vi "MegaAwesome_8_30_12a_JW.vi"() -> ()   [LabVIEW 2011]
uses:
  MegaAwesome_States.ctl
  <vilib>/Utility/file.llb/Read From Spreadsheet File (string).vi
  <vilib>/Utility/file.llb/Write To Spreadsheet File (string).vi
panel:
  in  "Slider Min":dbl=5.0
  in  "Slider Max":dbl=5.0
  out "Opj X Axis":string
  out "X Axis Display Type":string
  in  "Index-Sat":dbl=5.0
  in  "Index-Lin":dbl=5.0
  in  "IndexLog-Lin":dbl=5.0
  in  "IndexLog-Sat":dbl=5.0 caption="Num Pts"
  out "Lin Id-Log Used":dbl[](array[numeric])
  out "Lin-Vg Array-Log Used":dbl[](array[numeric])
  out "Total Width":dbl
  in  "New: Comments":string
  out "Save Array":string[][](array[string])
  out "Folder Index":i32 caption="Length"
  out "Sat Id-Used":dbl[](array[numeric])
  out "Sat Vg Array-Used":dbl[](array[numeric])
  out "Vg Array-Log-Used":dbl[](array[numeric])
  out "Sat Id-Log-Used":dbl[](array[numeric])
  out "Lin Id-Used":dbl[](array[numeric])
  out "Lin-Vg Array-Used":dbl[](array[numeric])
  out "Lin Vd":dbl
  out "Recorded Prop":T1
  out "Current State":T2
  in  "Main Tab Control":T3(tab)
  in  "Image Folder":path
  out "Image File":path=path "D:/UserData/Desktop/Jeremy/WFU/Research/Programs/VI mods/Image Not Found.png"
  in  "Transfer File":path
  out "Transfer Folder":path
  out "Fabrication Prop":T4
  in  "Transfer Plots":T5(tab)=enum."Saturation"
  in  "Lin-Trans Slider":dbl(slide) step=1.0 scale=-40.0..40.0 scale format="%#_1p"
  out "Sqrt-Lin":cluster{dbl[], dbl[]}[](graph)
  in  "Sat-Trans Slider":dbl(slide) step=1.0 scale=-40.0..40.0 scale format="%#_1p"
  out "Sqrt-Sat":cluster{dbl[], dbl[]}[](graph)
  out "Raw- Lin":cluster{dbl[], dbl[]}[](graph)
  out "Raw- Sat":cluster{dbl[], dbl[]}[](graph)
  in  "Log Plots":enum32{"Linear", "Saturation", "Transport"}(tab)=enum."Saturation"
  in  "Lin-Log Slider":dbl(slide) step=1.0 scale=-40.0..40.0 scale format="%#_1p"
  out "Log-Lin":cluster{dbl[], dbl[]}[](graph)
  in  "Sat-Log Slider":dbl(slide) step=1.0 scale=-40.0..40.0 scale format="%#_1p"
  out "Sat-Log":cluster{dbl[], dbl[]}[](graph)
  out "Transport":cluster{dbl[], dbl[]}[](graph)
  in  "Manual Controls":T6
  in  "File Controls":T7
  out "Date Recorded":string="Date Recorded" caption="Measured"
  out "Data Name:":string
  out "Image Name":string
  out "Index":string
  out "Date Created":string caption="Fabricated"
  in  "Comments:":string
  out "Rec: Length":dbl caption="Length" format="%#_3g"
  out "Rec: Width":dbl caption="Width" format="%#_4g"
  out "Rec: Dielectric (d)":dbl caption="Dielectric (d)" format="%#_3g"
  in  "New: Dielectric":dbl
  in  "New: Length":dbl
  in  "New: Width":dbl
  out "Rec: Temp":dbl caption="Sample Temp" format="%.1f"
  in  "New: Temp":dbl format="%.1f"
  out "Image Out":T8(plugin-control)
  in  "Num Pts":dbl=5.0
  in  "Num Pts Log":dbl=5.0 caption="Num Pts"
  out "Recorded Values Cluster":T9
  out "Calculated Values Cluster":T9 caption="Recorded Values Cluster"
  out "Re-Calculated Values Cluster":T9 caption="Recorded Values Cluster"
  in  "Independant Variable:":string(combo)="Length (um):"
  out "Image Preview":T8(plugin-control)
  in  "No Image File":path=path "\\\\acad1\\physics/Jurchescu-group/JW-PD/Mega Awesome/Image Not Found.png"
  in  "Room Temp":dbl=294.0
  in  "Origin Project File":path=path "\\\\acad1\\physics/Jurchescu-group/JW-PD/Group Library/Origin Project Files/DeviceData_8_10_12a_JW.opj"
  in  "Transport Style Controls":T10={"Transport Line Size"=1, "Transport Line Color"=16772608} {"Transport Line Size" items=["Extra Small", "Small", "Medium", "Large", "Extra Large"]}
  # "Image Location"
  # "Recorded"
  # "Calculated"
  # "Re-Calculated"
  # "Manual"
  # "Used points display at y=0\nValues are wrong w/ slider"
  # "Slider\nDoesn't\nWork"
  # "Slider\nDoesn't\nWork"
  # "No new points displayed"
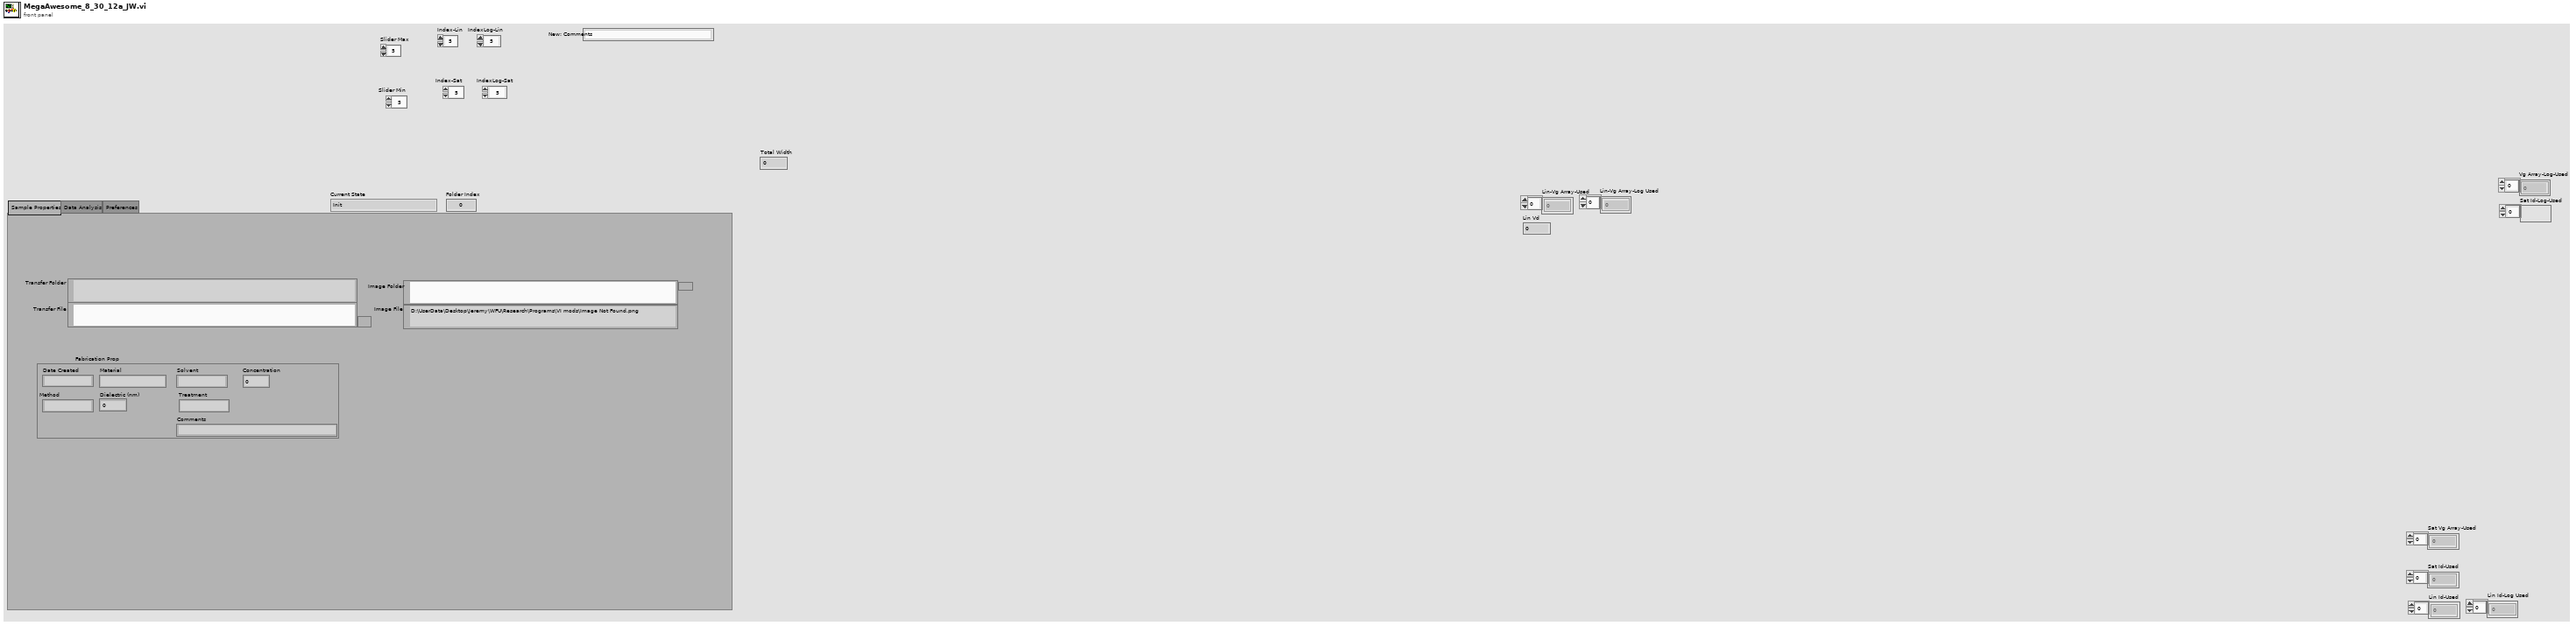
[diagram p1: front panel]
types:
  T1 = cluster{"Date Recorded":string, "Index":string, "Length":dbl, "Width":dbl, "Sample Temp":dbl}
  T2 = typedef "MegaAwesome_States.ctl" = enum16{"Init", "File Missing", "No Event", "Read Data", "Calculated Values", "Re-Calculated Values", "Next File", "Previous File", "Discard File", "Save", "Save Lines", "Export", "Exit"}
  T3 = enum32{"Sample Properties", "Data Analysis", "Preferences"}
  T4 = cluster{"Date Created":string, "Material":string, "Solvent":string, "Concentration":dbl, "Method":string, "Dielectric (nm)":dbl, "Treatment":string, "Comments":string}
  T5 = enum32{"Linear", "Saturation", "Raw-Linear", "Raw-Saturation"}
  T6 = cluster{"Manual-Temp":bool, "Manual-Width":bool, "Manuel-Length":bool, "Manuel-Dielectric":bool, "Manual Comments":bool}
  T7 = cluster{"Previous File":bool, "Discard ":bool, "Save Lines":bool, "Close":bool, "Next File ":bool, "Save":bool, "Save Next":bool, "Export":bool}
  T8 = typedef "IMAQ Image.ctl" = refnum<image>
  T9 = cluster{"Mobility-Sat":dbl, "Moblitity-Lin":dbl, "On/Off":dbl, "Off Current":dbl, "Vt-Sat":dbl, "STS":dbl, "Trap Density-VT":dbl, "Trap Density-STS":dbl}
  T10 = cluster{"Transport Line Size":u16, "Transport Line Color":u32}
  T11 = cluster{"[0]":cluster{dbl[], dbl[]}, "[1]":cluster{dbl[], dbl[]}, "[2]":cluster{dbl[], dbl[]}, "[3]":cluster{dbl[], dbl[]}, "[4]":cluster{dbl[], dbl[]}, "[5]":cluster{dbl[], dbl[]}, "[6]":cluster{dbl[], dbl[]}, "[7]":cluster{dbl[], dbl[]}, "[8]":cluster{dbl[], dbl[]}}
  T12 = cluster{"Sat Vg Used":dbl[], "Sat Sqrt(Id) Used ":dbl[], "Lin Vg Used":dbl[], "Lin Sqrt(Id) Used":dbl[], "Index-Lin":dbl, "Index-Sat":dbl}
  T13 = cluster{"Raw Sat":cluster{dbl[], dbl[]}[], "Sqrt Sat":cluster{dbl[], dbl[]}[], "Log Sat":cluster{dbl[], dbl[]}[], "Raw Lin":cluster{dbl[], dbl[]}[], "Sqrt Lin":cluster{dbl[], dbl[]}[], "Log Lin":cluster{dbl[], dbl[]}[]}
  T14 = cluster{"Mobility-Sat":dbl, "Vt-Sat":dbl, "Mobility-Lin":dbl, "Vt-Lin":dbl, "Off I-Sat":dbl, "On/Off I-Sat":dbl}
  T15 = cluster{"Sat Vg Used":dbl[], "Sat Log(Id) Used":dbl[], "Lin Vg Used":dbl[], "Lin Log(Id) Used":dbl[], "STS Index-Sat":dbl, "STS Index-Lin":dbl}
  T16 = cluster{"Independant  Variable Indicator":string, "Parameter String Indicator":string}
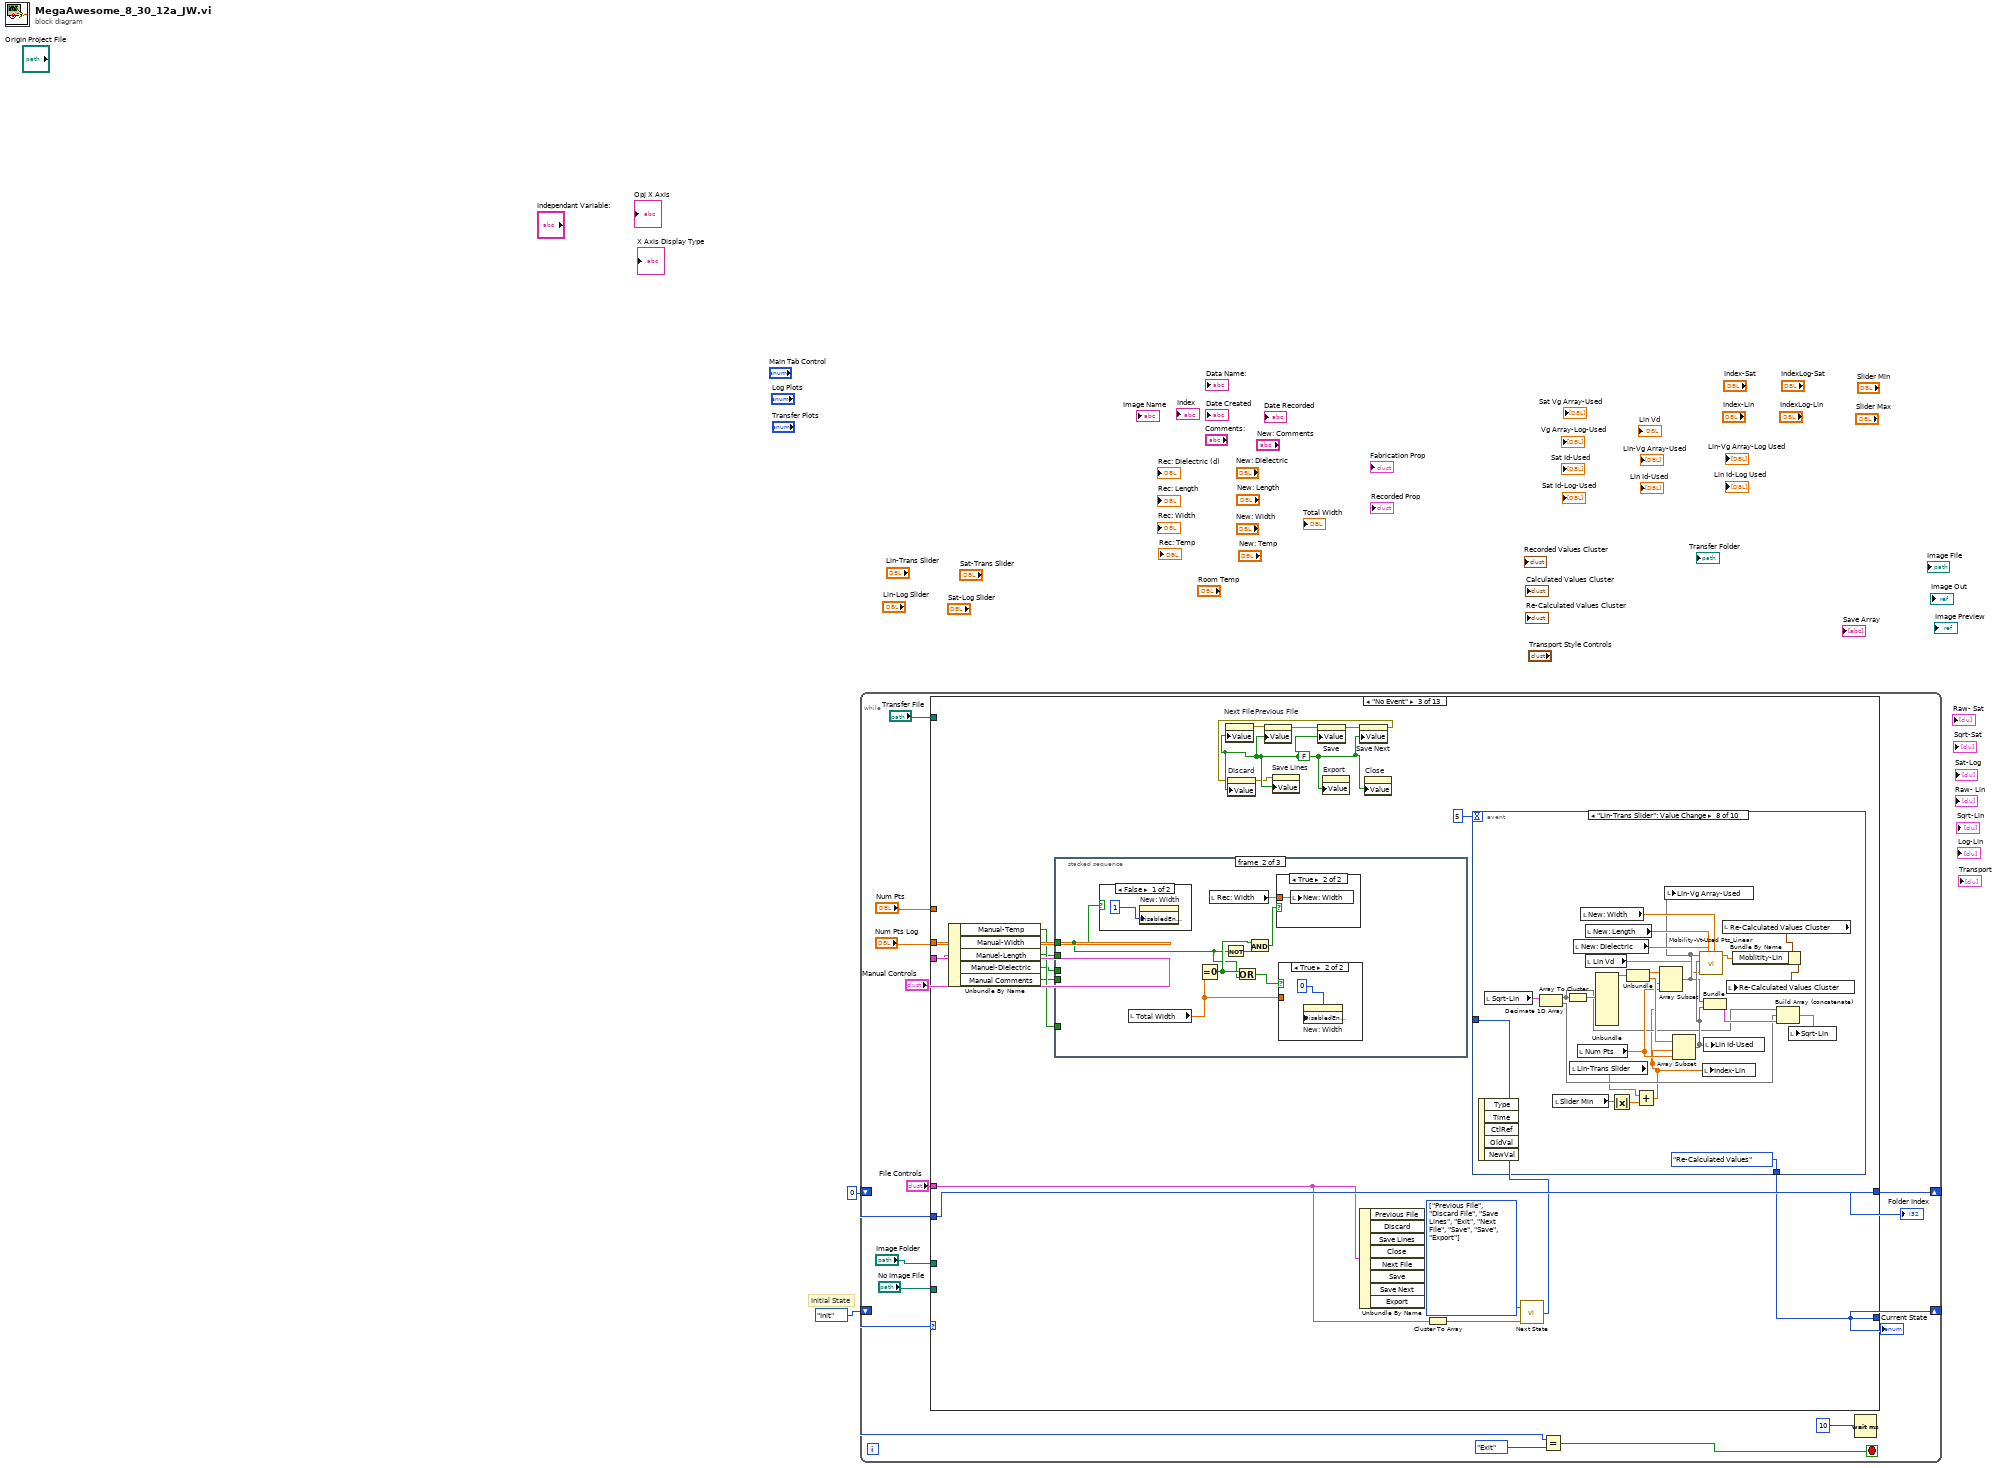
[diagram p0: block diagram]
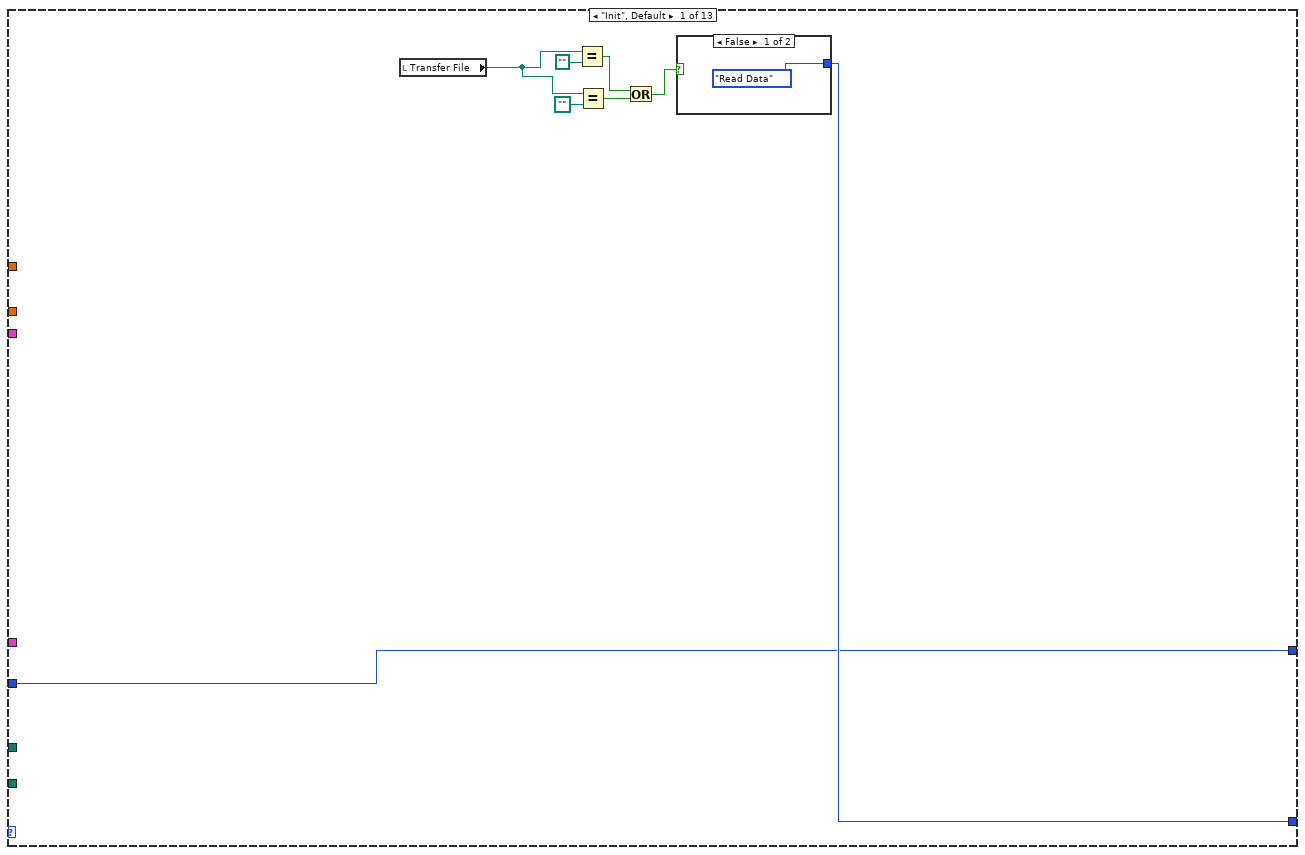
[diagram p2: hidden frame]
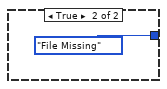
[diagram p3: hidden frame]
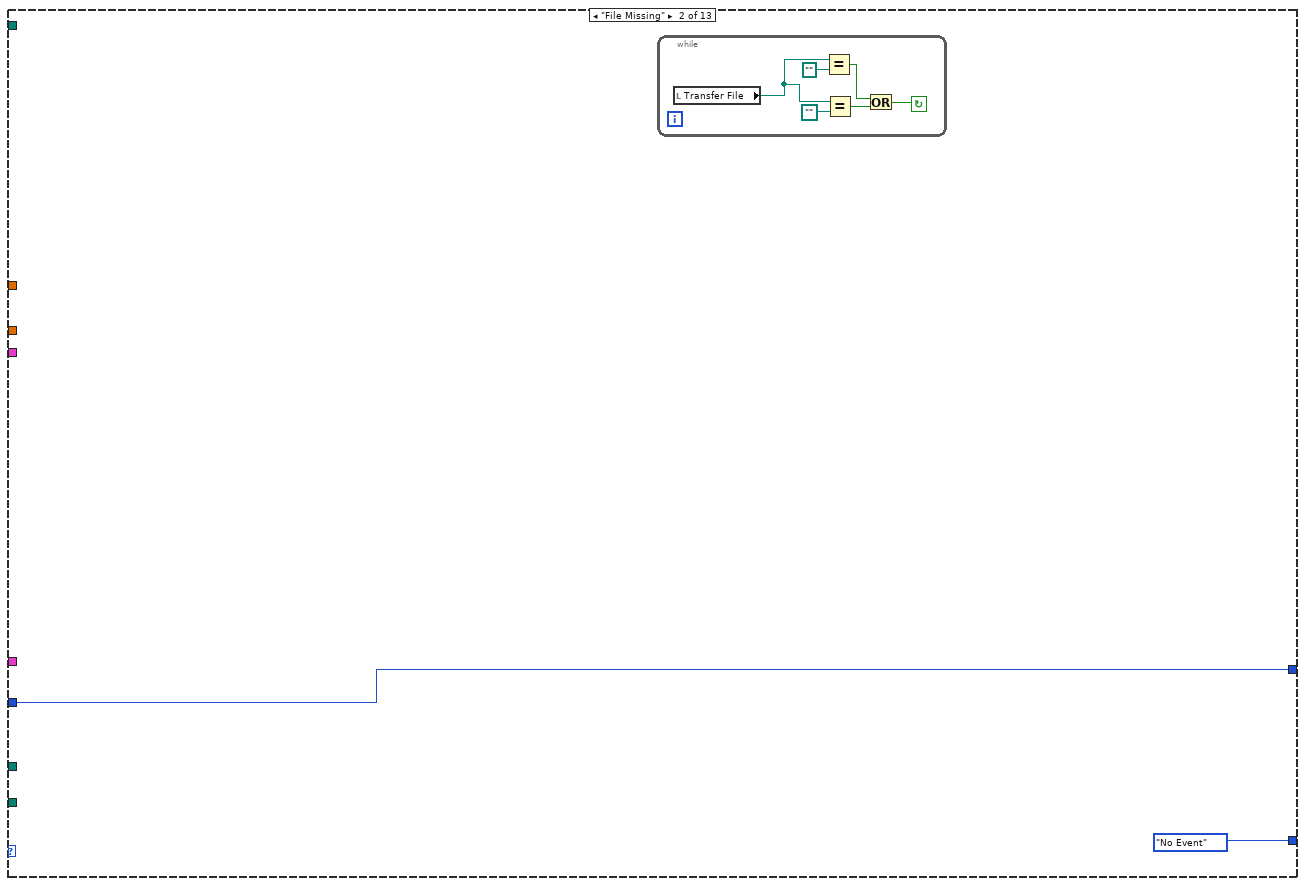
[diagram p4: hidden frame]
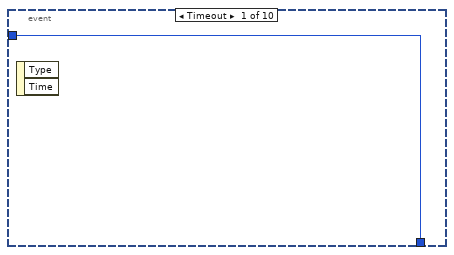
[diagram p5: hidden frame]
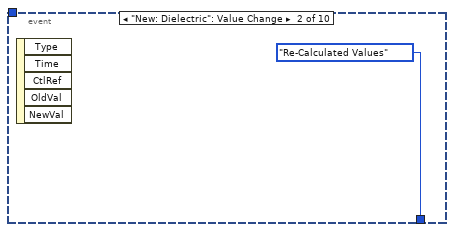
[diagram p6: hidden frame]
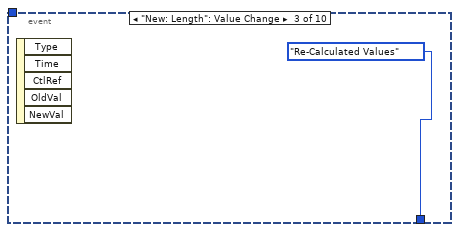
[diagram p7: hidden frame]
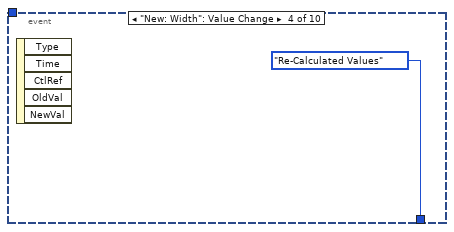
[diagram p8: hidden frame]
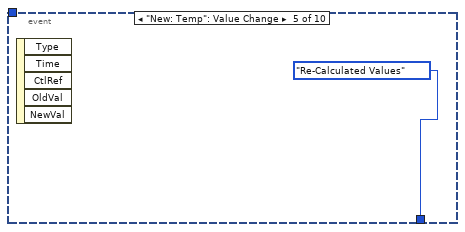
[diagram p9: hidden frame]
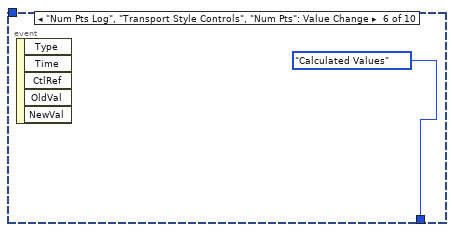
[diagram p10: hidden frame]
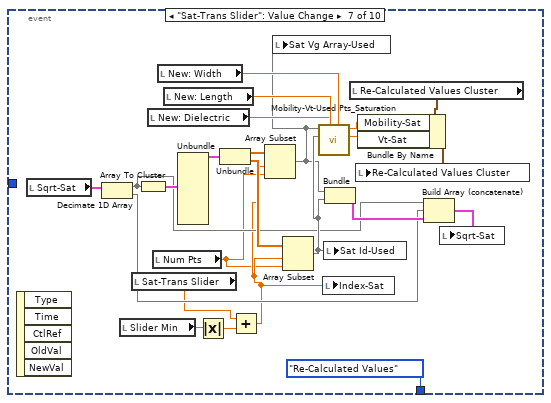
[diagram p11: hidden frame]
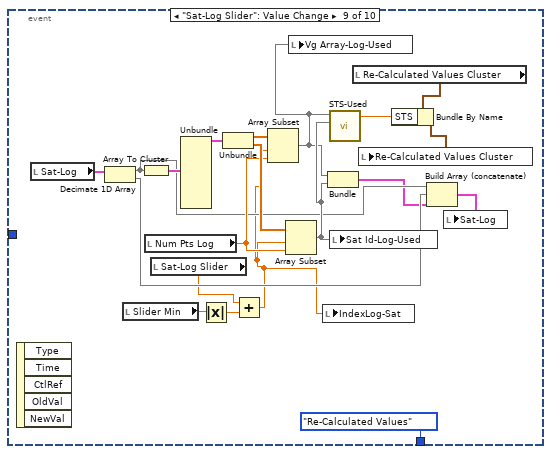
[diagram p12: hidden frame]
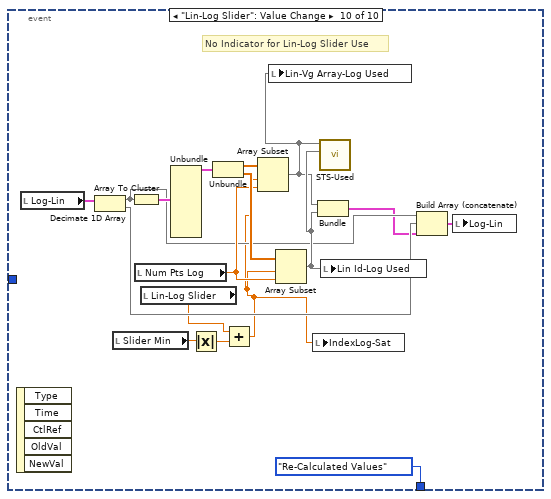
[diagram p13: hidden frame]
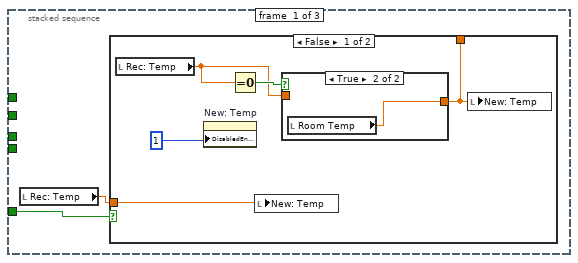
[diagram p14: hidden frame]
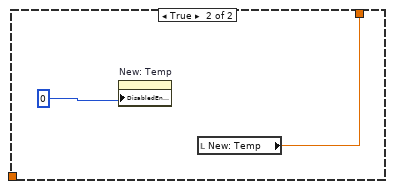
[diagram p16: hidden frame]
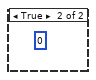
[diagram p17: hidden frame]
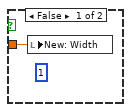
[diagram p19: hidden frame]
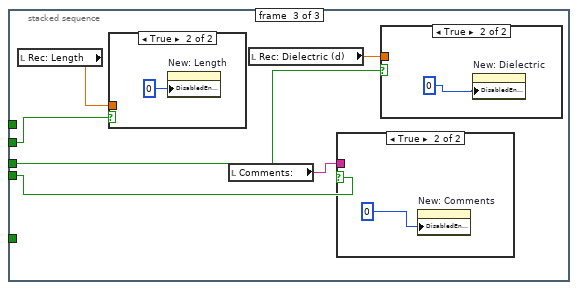
[diagram p20: hidden frame]
diagram:
  # "Initial State"
  n1 = while {
    shift-right: [w13] -> _
    shift-left: MegaAwesome_States."Init" -> [w15]
    shift-right: [w6] -> _
    shift-left: 0 -> [w7]
    stop <- w16 stop-if-true
    n2 = case shown="\"No Event\"" w15 {
      tunnel: [w18 MegaAwesome_States."No Event" w43 MegaAwesome_States."Calculated Values" MegaAwesome_States."Re-Calculated Values" MegaAwesome_States."No Event" MegaAwesome_States."Read Data" MegaAwesome_States."Read Data" MegaAwesome_States."No Event" w341 MegaAwesome_States."No Event" MegaAwesome_States."No Event" MegaAwesome_States."Exit"] -> w13
      tunnel: "Transfer File" -> [_ _ _ w188 w225 _ w310 w322 _ w346 _ _ _]
      tunnel: "Num Pts" -> [_ _ _ _ w249 _ _ _ _ _ _ _ _]
      tunnel: "Num Pts Log" -> [_ _ _ _ w248 _ _ _ _ _ _ _ _]
      tunnel: "Image Folder" -> [_ _ _ _ w245 _ _ _ _ _ _ _ _]
      tunnel: "No Image File" -> [_ _ _ _ w244 _ _ _ _ _ _ _ _]
      tunnel: [w17 w27 w51 w182 w243 w270 w295 w320 w338 w347 w862 w865 w866] -> w6
      tunnel: w7 -> [w17 w27 w51 _ w243 w270 w296 w321 w338 w347 w862 w865 w866]
      tunnel: "Manual Controls" -> [_ _ w45 _ _ _ _ _ _ w345 _ _ _]
      tunnel: "File Controls" -> [_ _ w41 _ _ _ _ _ _ w340 _ _ _]
      frame "Init", Default {
        n3 = local read "Transfer File"() -> (w19:path)
        n4 = Equal?(x=w19, y=path "") -> (x = y?=w22:bool)
        n5 = Equal?(x=w19, y=path "") -> (x = y?=w21:bool)
        n6 = Or(x=w22, y=w21) -> (x .or. y?=w24:bool)
        n7 = case shown="False" w24 {
          tunnel: [MegaAwesome_States."Read Data" MegaAwesome_States."File Missing"] -> w18
          frame False {
          }
          frame True {
          }
        }
      }
      frame "File Missing" {
        n8 = while {
          stop <- w29 continue-if-true
          n9 = local read "Transfer File"() -> (w30:path)
          n10 = Equal?(x=w30, y=path "") -> (x = y?=w32:bool)
          n11 = Equal?(x=w30, y=path "") -> (x = y?=w33:bool)
          n12 = Or(x=w32, y=w33) -> (x .or. y?=w29:bool)
        }
      }
      frame "No Event" {
        w40 = FALSE
        w53 = T2[] [enum."Previous File", enum."Discard File", enum."Save Lines", enum."Exit", enum."Next File", enum."Save", enum."Save", enum."Export"] items=["Init", "File Missing", "No Event", "Read Data", "Calculated Values", "Re-Calculated Values", "Next File", "Previous File", "Discard File", "Save", "Save Lines", "Export", "Exit"]
        n13 = Unbundle By Name(w45) -> ("Manual-Temp"=w50:bool, "Manual-Width"=w49:bool, "Manuel-Length"=w48:bool, "Manuel-Dielectric"=w47:bool, "Manual Comments"=w46:bool)
        n14 = stacked-sequence {
          tunnel: w50 -> [w146 _ _]
          tunnel: w49 -> [_ w156 _]
          tunnel: w48 -> [_ _ w171]
          tunnel: w47 -> [_ _ w168]
          tunnel: w46 -> [_ _ w167]
          frame #0 {
            n15 = local read "Rec: Temp"() -> (w145:dbl)
            n16 = case shown="False" w146 {
              tunnel: w145 -> [w151 _]
              tunnel: [w148 w155] -> _
              frame False {
                n17 = local read "Rec: Temp"() -> (w149:dbl)
                n18 = property on="New: Temp" class="DigNum (strict)"("DisabledEnum"=1) -> ()  [unwired: 2 in, 2 out]
                n19 = Equal To 0?(x=w149) -> (x = 0?=w150:bool)
                n20 = local write "New: Temp"(w151) -> ()
                n21 = case shown="True" w150 {
                  tunnel: [w152 w153] -> w148
                  tunnel: w149 -> [w152 _]
                  frame False {
                  }
                  frame True {
                    n22 = local read "Room Temp"() -> (w153:dbl)
                  }
                }
                n23 = local write "New: Temp"(w148) -> ()
              }
              frame True {
                n24 = property on="New: Temp" class="DigNum (strict)"("DisabledEnum"=0) -> ()  [unwired: 2 in, 2 out]
                n25 = local read "New: Temp"() -> (w155:dbl)
              }
            }
          }
          frame #1 {
            n26 = case shown="False" w156 {
              frame False {
                n27 = property on="New: Width" class="DigNum (strict)"("DisabledEnum"=1) -> ()  [unwired: 2 in, 2 out]
              }
              frame True {
                (unwired) 0
              }
            }
            n28 = local read "Total Width"() -> (w162:dbl)
            n29 = Equal To 0?(x=w162) -> (x = 0?=w159:bool)
            n30 = local read "Rec: Width"() -> (w160:dbl)
            n31 = Not(x=w156) -> (.not. x?=w158:bool)
            n32 = Or(x=w159, y=w156) -> (x .or. y?=w161:bool)
            n33 = And(x=w159, y=w158) -> (x .and. y?=w157:bool)
            n34 = case shown="True" w157 {
              tunnel: w160 -> [_ w164]
              frame False {
              }
              frame True {
                n35 = local write "New: Width"(w164) -> ()
              }
            }
            n36 = case shown="True" w161 {
              tunnel: w162 -> [w165 _]
              frame False {
                (unwired) 1
                n37 = local write "New: Width"(w165) -> ()
              }
              frame True {
                n38 = property on="New: Width" class="DigNum (strict)"("DisabledEnum"=0) -> ()  [unwired: 2 in, 2 out]
              }
            }
          }
          frame #2 {
            n39 = local read "Rec: Length"() -> (w172:dbl)
            n40 = case shown="True" w171 {
              tunnel: w172 -> [w180 _]
              frame False {
                n41 = local write "New: Length"(w180) -> ()
                n42 = property on="New: Length" class="DigNum (strict)"("DisabledEnum"=1) -> ()  [unwired: 2 in, 2 out]
              }
              frame True {
                n43 = property on="New: Length" class="DigNum (strict)"("DisabledEnum"=0) -> ()  [unwired: 2 in, 2 out]
              }
            }
            n44 = local read "Comments:"() -> (w169:string)
            n45 = local read "Rec: Dielectric (d)"() -> (w170:dbl)
            n46 = case shown="True" w167 {
              tunnel: w169 -> [w174 _]
              frame False {
                n47 = local write "New: Comments"(w174) -> ()
                n48 = property on="New: Comments" class="Str"("DisabledEnum"=1) -> ()  [unwired: 2 in, 2 out]
              }
              frame True {
                n49 = property on="New: Comments" class="Str"("DisabledEnum"=0) -> ()  [unwired: 2 in, 2 out]
              }
            }
            n50 = case shown="True" w168 {
              tunnel: w170 -> [w177 _]
              frame False {
                n51 = local write "New: Dielectric"(w177) -> ()
                n52 = property on="New: Dielectric" class="DigNum (strict)"("DisabledEnum"=1) -> ()  [unwired: 2 in, 2 out]
              }
              frame True {
                n53 = property on="New: Dielectric" class="DigNum (strict)"("DisabledEnum"=0) -> ()  [unwired: 2 in, 2 out]
              }
            }
          }
        }
        n54 = property on="Next File" class="Bool (strict)"("Value"=w40) -> (error out=w39:errorcluster)  [unwired: 2 in, 1 out]
        n55 = property on="Previous File" class="Bool (strict)"(error in=w39, "Value"=w40) -> (error out=w38:errorcluster)  [unwired: 1 in, 1 out]
        n56 = property on="Save" class="Bool (strict)"(error in=w38, "Value"=w40) -> (error out=w37:errorcluster)  [unwired: 1 in, 1 out]
        n57 = property on="Export" class="Bool (strict)"("Value"=w40) -> ()  [unwired: 2 in, 2 out]
        n58 = Unbundle By Name(w41) -> ()  [unwired: 8 out]
        n59 = property on="Save Next" class="Bool (strict)"(error in=w37, "Value"=w40) -> (error out=w36:errorcluster)  [unwired: 1 in, 1 out]
        n60 = property on="Discard" class="Bool (strict)"(error in=w36, "Value"=w40) -> (error out=w35:errorcluster)  [unwired: 1 in, 1 out]
        n61 = property on="Save Lines" class="Bool (strict)"(error in=w35, "Value"=w40) -> ()  [unwired: 1 in, 2 out]
        n62 = property on="Close" class="Bool (strict)"("Value"=w40) -> ()  [unwired: 2 in, 2 out]
        n63 = Cluster To Array(cluster=w41) -> (array=w52:bool[])
        n64 = call "Next State.vi"("Buttons []"=w52, "States []"=w53) -> ("Enum"=w44:T2)
        n65 = event shown="[7] \"Lin-Trans Slider\": Value Change" {
          selector: _ -> [_ _ _ _ _ _ _ _ _ _]
          dyn-events: _ -> [_ _ _ _ _ _ _ _ _ _]
          timeout: 5 -> [_ _ _ _ _ _ _ _ _ _]
          tunnel: w44 -> [w54 _ _ _ _ _ _ _ _ _]
          tunnel: [w54 MegaAwesome_States."Re-Calculated Values" MegaAwesome_States."Re-Calculated Values" MegaAwesome_States."Re-Calculated Values" MegaAwesome_States."Re-Calculated Values" MegaAwesome_States."Calculated Values" MegaAwesome_States."Re-Calculated Values" MegaAwesome_States."Re-Calculated Values" MegaAwesome_States."Re-Calculated Values" MegaAwesome_States."Re-Calculated Values"] -> w43
          event Timeout {
            n66 = event-data() -> ()  [unwired: 1 in, 2 out]
          }
          event "New: Dielectric": Value Change {
            n67 = event-data() -> ()  [unwired: 1 in, 5 out]
          }
          event "New: Length": Value Change {
            n68 = event-data() -> ()  [unwired: 1 in, 5 out]
          }
          event "New: Width": Value Change {
            n69 = event-data() -> ()  [unwired: 1 in, 5 out]
          }
          event "New: Temp": Value Change {
            n70 = event-data() -> ()  [unwired: 1 in, 5 out]
          }
          event "Num Pts Log", "Transport Style Controls", "Num Pts": Value Change {
            n71 = event-data() -> ()  [unwired: 1 in, 5 out]
          }
          event "Sat-Trans Slider": Value Change {
            n72 = event-data() -> ()  [unwired: 1 in, 5 out]
            n73 = local read "Sqrt-Sat"() -> (w83:cluster{dbl[], dbl[]}[])
            n74 = Decimate 1D Array(w83) -> (w67:cluster{dbl[], dbl[]}[], w68:cluster{dbl[], dbl[]}[])
            n75 = local read "Slider Min"() -> (w64:dbl)
            n76 = local read "Sat-Trans Slider"() -> (w62:dbl)
            n77 = Array To Cluster(array=w67) -> (cluster=w82:T11)
            n78 = local read "New: Dielectric"() -> (w77:dbl)
            n79 = local read "Num Pts"() -> (w60:dbl)
            n80 = local read "New: Width"() -> (w79:dbl)
            n81 = local read "New: Length"() -> (w78:dbl)
            n82 = Unbundle(w82) -> ("[0]"=w81:cluster{dbl[], dbl[]})  [unwired: 8 out]
            n83 = Absolute Value(x=w64) -> (abs(x)=w63:dbl)
            n84 = Unbundle(w81) -> (w65:dbl[], w80:dbl[])
            n85 = Add(x=w62, y=w63) -> (x+y=w61:dbl)
            n86 = Array Subset(array=w65, index=w61, length=w60) -> (w75:dbl[])
            n87 = local write "Sat Vg Array-Used"(w75) -> ()
            n88 = Array Subset(array=w80, index=w61, length=w60) -> (w76:dbl[])
            n89 = call "Mobility-Vt-Used Pts_Saturation.vi"("Width"=w79, "Length"=w78, "Dielectric (d)"=w77, "Sat Id Used"=w76, "Vg Used"=w75) -> ("Vt"=w71:dbl, "Mobility"=w72:dbl)  [unwired: 4 in, 1 out]
            n90 = local write "Index-Sat"(w61) -> ()
            n91 = local write "Sat Id-Used"(w76) -> ()
            n92 = Bundle(w75, w76) -> (w69:cluster{dbl[], dbl[]})  [unwired: 1 in]
            n93 = local read "Re-Calculated Values Cluster"() -> (w74:T9)
            n94 = Bundle By Name(cluster=w74, "Mobility-Sat"=w72, "Vt-Sat"=w71) -> (w73:T9)
            n95 = local write "Re-Calculated Values Cluster"(w73) -> ()
            n96 = Build Array (concatenate)(w67, w68, w69) -> (w66:cluster{dbl[], dbl[]}[])
            n97 = local write "Sqrt-Sat"(w66) -> ()
          }
          event "Lin-Trans Slider": Value Change {
            n98 = event-data() -> ()  [unwired: 1 in, 5 out]
            n99 = local read "Sqrt-Lin"() -> (w107:cluster{dbl[], dbl[]}[])
            n100 = Decimate 1D Array(w107) -> (w92:cluster{dbl[], dbl[]}[], w93:cluster{dbl[], dbl[]}[])
            n101 = local read "Slider Min"() -> (w89:dbl)
            n102 = Array To Cluster(array=w92) -> (cluster=w106:T11)
            n103 = local read "Lin-Trans Slider"() -> (w87:dbl)
            n104 = local read "New: Dielectric"() -> (w100:dbl)
            n105 = local read "Num Pts"() -> (w103:dbl)
            n106 = local read "New: Width"() -> (w102:dbl)
            n107 = local read "New: Length"() -> (w101:dbl)
            n108 = local read "Lin Vd"() -> (w84:dbl)
            n109 = Unbundle(w106) -> ("[0]"=w105:cluster{dbl[], dbl[]})  [unwired: 8 out]
            n110 = Absolute Value(x=w89) -> (abs(x)=w88:dbl)
            n111 = Unbundle(w105) -> (w90:dbl[], w104:dbl[])
            n112 = Add(x=w87, y=w88) -> (x+y=w86:dbl)
            n113 = Array Subset(array=w90, index=w86, length=w103) -> (w98:dbl[])
            n114 = local write "Lin-Vg Array-Used"(w98) -> ()
            n115 = Array Subset(array=w104, index=w86, length=w103) -> (w99:dbl[])
            n116 = call "Mobility-Vt-Used Pts_Linear.vi"("Width"=w102, "Length"=w101, "Vd"=w84, "Dielectric (d)"=w100, "Id Used"=w99, "Vg Used"=w98) -> ("Mobility"=w95:dbl)  [unwired: 3 in, 2 out]
            n117 = local write "Index-Lin"(w86) -> ()
            n118 = local write "Lin Id-Used"(w99) -> ()
            n119 = Bundle(w98, w99) -> (w94:cluster{dbl[], dbl[]})  [unwired: 1 in]
            n120 = local read "Re-Calculated Values Cluster"() -> (w97:T9)
            n121 = Bundle By Name(cluster=w97, "Moblitity-Lin"=w95) -> (w96:T9)
            n122 = local write "Re-Calculated Values Cluster"(w96) -> ()
            n123 = Build Array (concatenate)(w92, w93, w94) -> (w91:cluster{dbl[], dbl[]}[])
            n124 = local write "Sqrt-Lin"(w91) -> ()
          }
          event "Sat-Log Slider": Value Change {
            n125 = event-data() -> ()  [unwired: 1 in, 5 out]
            n126 = local read "Sat-Log"() -> (w110:cluster{dbl[], dbl[]}[])
            n127 = Decimate 1D Array(w110) -> (w117:cluster{dbl[], dbl[]}[], w118:cluster{dbl[], dbl[]}[])
            n128 = local read "Slider Min"() -> (w114:dbl)
            n129 = Array To Cluster(array=w117) -> (cluster=w127:T11)
            n130 = local read "Num Pts Log"() -> (w124:dbl)
            n131 = local read "Sat-Log Slider"() -> (w112:dbl)
            n132 = Unbundle(w127) -> ("[0]"=w126:cluster{dbl[], dbl[]})  [unwired: 8 out]
            n133 = Absolute Value(x=w114) -> (abs(x)=w113:dbl)
            n134 = Unbundle(w126) -> (w115:dbl[], w125:dbl[])
            n135 = Add(x=w112, y=w113) -> (x+y=w109:dbl)
            n136 = Array Subset(array=w115, index=w109, length=w124) -> (w122:dbl[])
            n137 = Array Subset(array=w125, index=w109, length=w124) -> (w123:dbl[])
            n138 = local write "Vg Array-Log-Used"(w122) -> ()
            n139 = local write "IndexLog-Sat"(w109) -> ()
            n140 = Bundle(w122, w123) -> (w108:cluster{dbl[], dbl[]})  [unwired: 1 in]
            n141 = call "STS-Used.vi"("Id Used"=w123, "Vg-Used"=w122) -> ("STS"=w119:dbl)  [unwired: 9 in]
            n142 = local write "Sat Id-Log-Used"(w123) -> ()
            n143 = local read "Re-Calculated Values Cluster"() -> (w121:T9)
            n144 = Bundle By Name(cluster=w121, "STS"=w119) -> (w120:T9)
            n145 = local write "Re-Calculated Values Cluster"(w120) -> ()
            n146 = Build Array (concatenate)(w117, w118, w108) -> (w116:cluster{dbl[], dbl[]}[])
            n147 = local write "Sat-Log"(w116) -> ()
          }
          event "Lin-Log Slider": Value Change {
            # "No Indicator for Lin-Log Slider Use"
            n148 = event-data() -> ()  [unwired: 1 in, 5 out]
            n149 = local read "Log-Lin"() -> (w131:cluster{dbl[], dbl[]}[])
            n150 = Decimate 1D Array(w131) -> (w137:cluster{dbl[], dbl[]}[], w138:cluster{dbl[], dbl[]}[])
            n151 = local read "Slider Min"() -> (w134:dbl)
            n152 = Array To Cluster(array=w137) -> (cluster=w144:T11)
            n153 = local read "Num Pts Log"() -> (w141:dbl)
            n154 = local read "Lin-Log Slider"() -> (w132:dbl)
            n155 = Unbundle(w144) -> ("[0]"=w143:cluster{dbl[], dbl[]})  [unwired: 8 out]
            n156 = Absolute Value(x=w134) -> (abs(x)=w133:dbl)
            n157 = Unbundle(w143) -> (w135:dbl[], w142:dbl[])
            n158 = Add(x=w132, y=w133) -> (x+y=w130:dbl)
            n159 = Array Subset(array=w135, index=w130, length=w141) -> (w139:dbl[])
            n160 = local write "Lin-Vg Array-Log Used"(w139) -> ()
            n161 = Array Subset(array=w142, index=w130, length=w141) -> (w140:dbl[])
            n162 = local write "IndexLog-Sat"(w130) -> ()
            n163 = Bundle(w139, w140) -> (w129:cluster{dbl[], dbl[]})  [unwired: 1 in]
            n164 = call "STS-Used.vi"("Id Used"=w140, "Vg-Used"=w139) -> ()  [unwired: 9 in, 1 out]
            n165 = local write "Lin Id-Log Used"(w140) -> ()
            n166 = Build Array (concatenate)(w137, w138, w129) -> (w136:cluster{dbl[], dbl[]}[])
            n167 = local write "Log-Lin"(w136) -> ()
          }
        }
      }
      frame "Read Data" {
        n168 = call "Recorded Values.vi"("Path"=w188) -> ("Recorded Char"=w206:T9, "Recorded Prop"=w196:T1, "Fabrication Prop"=w190:T4)  [unwired: 8 in]
        n169 = Strip Path(path=w188) -> (stripped path=w189:path, name=w187:string)
        n170 = local write "Fabrication Prop"(w190) -> ()
        n171 = local write "Recorded Prop"(w196) -> ()
        n172 = Unbundle By Name(w196) -> ("Date Recorded"=w195:string, "Index"=w193:string, "Length"=w194:dbl, "Width"=w192:dbl, "Sample Temp"=w191:dbl)
        n173 = local write "Recorded Values Cluster"(w206) -> ()
        n174 = Unbundle By Name(w196) -> ("Sample Temp"=w199:dbl)
        n175 = Unbundle By Name(w190) -> ("Dielectric (nm)"=w184:dbl, "Comments"=w183:string)
        n176 = List Folder(path=w189) -> (filenames=w185:string[])  [unwired: 3 in, 3 out]
        n177 = local write "Rec: Dielectric (d)"(w184) -> ()
        n178 = local write "Date Created"(w195) -> ()
        n179 = local write "Index"(w193) -> ()
        n180 = local write "Rec: Length"(w194) -> ()
        n181 = local write "Rec: Width"(w192) -> ()
        n182 = local write "Rec: Temp"(w191) -> ()
        n183 = Equal To 0?(x=w199) -> (x = 0?=w202:bool)
        n184 = Number To Decimal String(number=w199) -> (decimal integer string=w203:string)  [unwired: 1 in]
        n185 = local write "Comments:"(w183) -> ()
        n186 = Search 1D Array(1D array=w185, element=w187) -> (index of element=w182:i32)  [unwired: 1 in]
        n187 = Equal?(x="", y=w203) -> (x = y?=w201:bool)
        n188 = Index Array(array=w185, index=w182) -> (element=w186:string)
        n189 = Or(x=w202, y=w201) -> (x .or. y?=w200:bool)
        n190 = local write "Data Name:"(w186) -> ()
        n191 = case shown="False" w200 {
          tunnel: [w207 w208] -> w197
          tunnel: w199 -> [w207 _]
          frame False {
          }
          frame True {
            n192 = local read "Room Temp"() -> (w208:dbl)
          }
        }
        n193 = local write "New: Temp"(w197) -> ()
        n194 = Bundle By Name(cluster=w196, "Sample Temp"=w197) -> (w198:T1)
        n195 = local write "Recorded Prop"(w198) -> ()
      }
      frame "Calculated Values" {
        n196 = local read "Transport Style Controls"() -> (w224:T10)
        n197 = local read "Fabrication Prop"() -> (w254:T4)
        n198 = local read "Recorded Prop"() -> (w247:T1)
        n199 = local read "Calculated Values Cluster"() -> (w264:T9)
        n200 = call "Mobility-Vt Calculator-File.vi"("NumPts"=w249, "Path"=w225) -> ("Used Points"=w242:T12, "Graph Cluster"=w231:T13, "Lin Vd"=w238:dbl, "Output"=w262:T14)  [unwired: 6 in]
        n201 = call "STS Calculator-File.vi"("NumPts"=w248, "Path"=w225) -> ("Used Points"=w236:T15, "XY Graph-Sat"=w215:cluster{dbl[], dbl[]}[], "XY Graph-Lin"=w216:cluster{dbl[], dbl[]}[], "Ouput"=w257:cluster{"STS-Sat":dbl, "STS-Lin":dbl})  [unwired: 6 in]
        n202 = call "TRF to TSP Plot.vi"("Transport Graph Properties"=w224, "Transfer File"=w225) -> ("Transport"=w223:cluster{ext[], ext[]}[])  [unwired: 7 in, 2 out]
        n203 = Array Size(array=w223) -> (size(s)=w222:i32)
        n204 = Unbundle By Name(w254) -> ("Dielectric (nm)"=w252:dbl)
        n205 = Unbundle By Name(w247) -> ("Sample Temp"=w246:dbl)
        n206 = Unbundle By Name(w262) -> ("Mobility-Sat"=w261:dbl, "Vt-Sat"=w253:dbl, "Mobility-Lin"=w260:dbl, "Off I-Sat"=w259:dbl, "On/Off I-Sat"=w258:dbl)  [unwired: 1 out]
        n207 = local write "Lin Vd"(w238) -> ()
        n208 = Unbundle By Name(w257) -> ("STS-Sat"=w251:dbl)  [unwired: 1 out]
        n209 = local write "Transport"(w223) -> ()
        n210 = for {
          N: w222 -> [_]
          tunnel: w224 -> [w268]
          i -> [w267]
          n211 = Unbundle By Name(w268) -> ("Transport Line Size"=w265:u16, "Transport Line Color"=w266:u32)
          n212 = property on="Transport" class="XYGraph (strict)"("Active Plot"=w267, "Plot.Plot Color"=w266, "Plot.Line Width"=w265) -> ()  [unwired: 2 in, 2 out]
        }
        n213 = local write "Sat-Log"(w215) -> ()
        n214 = local write "Log-Lin"(w216) -> ()
        n215 = call "Trap Density_VT.vi"("VT"=w253, "Dielectric"=w252) -> ("Trap Density-VT"=w256:dbl)
        n216 = call "Trap Density_STS.vi"("Temp (T) [K]"=w246, "S.T.S. (S)"=w251, "Dielectric"=w252) -> ("Trap Density (N)"=w255:dbl)  [unwired: 8 in]
        n217 = call "Image from TRF Display.vi"("No Image File"=w244, "Image Folder"=w245, "Transfer File"=w225) -> ("Image Out 2"=w209:T8, "Image Out"=w210:T8, "Image File"=w211:path, "Image Name"=w212:string)  [unwired: 5 in]
        n218 = Bundle By Name(cluster=w264, "Mobility-Sat"=w261, "Moblitity-Lin"=w260, "On/Off"=w258, "Off Current"=w259, "Vt-Sat"=w253, "STS"=w251, "Trap Density-VT"=w256, "Trap Density-STS"=w255) -> (w263:T9)
        n219 = Unbundle By Name(w236) -> ("Sat Vg Used"=w235:dbl[], "Sat Log(Id) Used"=w234:dbl[], "Lin Vg Used"=w233:dbl[], "Lin Log(Id) Used"=w232:dbl[], "STS Index-Sat"=w213:dbl, "STS Index-Lin"=w214:dbl)
        n220 = Unbundle By Name(w242) -> ("Sat Vg Used"=w241:dbl[], "Sat Sqrt(Id) Used"=w240:dbl[], "Lin Vg Used"=w239:dbl[], "Lin Sqrt(Id) Used"=w237:dbl[], "Index-Lin"=w227:dbl, "Index-Sat"=w226:dbl)
        n221 = local write "Image File"(w211) -> ()
        n222 = local write "Image Name"(w212) -> ()
        n223 = local write "Image Out"(w210) -> ()
        n224 = local write "Image Preview"(w209) -> ()
        n225 = local write "Vg Array-Log-Used"(w235) -> ()
        n226 = local write "Sat Id-Log-Used"(w234) -> ()
        n227 = local write "Lin-Vg Array-Log Used"(w233) -> ()
        n228 = local write "Lin Id-Log Used"(w232) -> ()
        n229 = local write "IndexLog-Sat"(w213) -> ()
        n230 = local write "Index-Lin"(w214) -> ()
        n231 = local write "Calculated Values Cluster"(w263) -> ()
        n232 = local write "Sat Vg Array-Used"(w241) -> ()
        n233 = local write "Sat Id-Used"(w240) -> ()
        n234 = local write "Lin-Vg Array-Used"(w239) -> ()
        n235 = local write "Lin Id-Used"(w237) -> ()
        n236 = local write "Index-Sat"(w226) -> ()
        n237 = local write "Index-Lin"(w227) -> ()
        n238 = local write "Lin-Log Slider"(w214) -> ()
        n239 = local write "Sat-Log Slider"(w213) -> ()
        n240 = local write "Sat-Trans Slider"(w226) -> ()
        n241 = local write "Lin-Trans Slider"(w227) -> ()
        n242 = Unbundle By Name(w231) -> ("Raw Sat"=w221:cluster{dbl[], dbl[]}[], "Sqrt Sat"=w228:cluster{dbl[], dbl[]}[], "Raw Lin"=w230:cluster{dbl[], dbl[]}[], "Sqrt Lin"=w229:cluster{dbl[], dbl[]}[])
        n243 = Index Array(array=w221) -> (element=w220:cluster{dbl[], dbl[]})  [unwired: 1 in]
        n244 = Unbundle(w220) -> (w219:dbl[])  [unwired: 1 out]
        n245 = Array Max & Min(array=w219) -> (max value=w218:dbl, min value=w217:dbl)  [unwired: 2 out]
        n246 = property on="Sat-Trans Slider" class="Slide (strict)"("Scale.Maximum"=w218, "Scale.Minimum"=w217) -> ()  [unwired: 2 in, 2 out]
        n247 = property on="Lin-Trans Slider" class="Slide (strict)"("Scale.Maximum"=w218, "Scale.Minimum"=w217) -> ()  [unwired: 2 in, 2 out]
        n248 = property on="Sat-Log Slider" class="Slide (strict)"("Scale.Maximum"=w218, "Scale.Minimum"=w217) -> ()  [unwired: 2 in, 2 out]
        n249 = property on="Lin-Log Slider" class="Slide (strict)"("Scale.Maximum"=w218, "Scale.Minimum"=w217) -> ()  [unwired: 2 in, 2 out]
        n250 = local write "Slider Max"(w218) -> ()
        n251 = local write "Slider Min"(w217) -> ()
        n252 = local write "Raw- Sat"(w221) -> ()
        n253 = local write "Raw- Lin"(w230) -> ()
        n254 = local write "Sqrt-Sat"(w228) -> ()
        n255 = local write "Sqrt-Lin"(w229) -> ()
      }
      frame "Re-Calculated Values" {
        n256 = local read "Vg Array-Log-Used"() -> (w277:dbl[])
        n257 = local read "Sat Vg Array-Used"() -> (w285:dbl[])
        n258 = local read "Lin-Vg Array-Used"() -> (w291:dbl[])
        n259 = local read "Sat Id-Log-Used"() -> (w276:dbl[])
        n260 = local read "New: Dielectric"() -> (w289:dbl)
        n261 = local read "New: Dielectric"() -> (w274:dbl)
        n262 = local read "New: Length"() -> (w288:dbl)
        n263 = local read "New: Length"() -> (w284:dbl)
        n264 = local read "New: Width"() -> (w287:dbl)
        n265 = local read "New: Width"() -> (w283:dbl)
        n266 = local read "Lin Id-Used"() -> (w290:dbl[])
        n267 = local read "Sat Id-Used"() -> (w282:dbl[])
        n268 = local read "Re-Calculated Values Cluster"() -> (w293:T9)
        n269 = local read "New: Dielectric"() -> (w273:dbl)
        n270 = local read "New: Temp"() -> (w272:dbl)
        n271 = local read "Lin Vd"() -> (w269:dbl)
        n272 = call "Mobility-Vt-Used Pts_Saturation.vi"("Width"=w283, "Length"=w284, "Dielectric (d)"=w274, "Sat Id Used"=w282, "Vg Used"=w285) -> ("Vt"=w280:dbl, "Mobility"=w281:dbl)  [unwired: 4 in, 1 out]
        n273 = call "STS-Used.vi"("Id Used"=w276, "Vg-Used"=w277) -> ("STS"=w275:dbl)  [unwired: 9 in]
        n274 = call "Mobility-Vt-Used Pts_Linear.vi"("Width"=w287, "Length"=w288, "Vd"=w269, "Dielectric (d)"=w289, "Id Used"=w290, "Vg Used"=w291) -> ("Mobility"=w286:dbl)  [unwired: 3 in, 2 out]
        n275 = call "Trap Density_VT.vi"("VT"=w280, "Dielectric"=w274) -> ("Trap Density-VT"=w279:dbl)
        n276 = call "Trap Density_STS.vi"("Temp (T) [K]"=w272, "S.T.S. (S)"=w275, "Dielectric"=w273) -> ("Trap Density (N)"=w271:dbl)  [unwired: 8 in]
        n277 = Bundle By Name(cluster=w293, "Mobility-Sat"=w281, "Moblitity-Lin"=w286, "Vt-Sat"=w280, "STS"=w275, "Trap Density-VT"=w279, "Trap Density-STS"=w271) -> (w292:T9)
        n278 = local write "Re-Calculated Values Cluster"(w292) -> ()
      }
      frame "Next File" {
        n279 = Strip Path(path=w310) -> (stripped path=w300:path, name=w308:string)
        n280 = local write "Transfer Folder"(w300) -> ()
        n281 = List Folder(path=w300) -> (filenames=w294:string[], error out=w303:errorcluster)  [unwired: 3 in, 2 out]
        n282 = Array Size(array=w294) -> (size(s)=w307:i32)
        n283 = Search 1D Array(1D array=w294, element=w308) -> (index of element=w305:i32)  [unwired: 1 in]
        n284 = Decrement(x=w307) -> (x-1=w306:i32)
        n285 = Equal?(x=w306, y=w305) -> (x = y?=w304:bool)
        n286 = case shown="False" w304 {
          tunnel: w296 -> [w313 _]
          tunnel: [w312 0] -> w295
          tunnel: w303 -> [w311 w314]
          tunnel: [w311 w314] -> _
          frame False {
            n287 = Increment(x=w313) -> (x+1=w312:i32)
          }
          frame True {
          }
        }
        n288 = Path To String(path=w300) -> (string=w301:string)
        n289 = Index Array(array=w294, index=w295) -> (element=w302:string)
        n290 = Concatenate Strings(w301, "\\", w302) -> (w298:string)
        n291 = String To Path(string=w298) -> (path=w297:path)
        n292 = local write "Transfer File"(w297) -> ()
      }
      frame "Previous File" {
        n293 = Strip Path(path=w322) -> (stripped path=w319:path, name=w331:string)
        n294 = local write "Transfer Folder"(w319) -> ()
        n295 = List Folder(path=w319) -> (filenames=w323:string[], error out=w328:errorcluster)  [unwired: 3 in, 2 out]
        n296 = Array Size(array=w323) -> (size(s)=w317:i32)
        n297 = Search 1D Array(1D array=w323, element=w331) -> (index of element=w330:i32)  [unwired: 1 in]
        n298 = Decrement(x=w317) -> (x-1=w316:i32)
        n299 = Equal To 0?(x=w330) -> (x = 0?=w329:bool)
        n300 = case shown="False" w329 {
          tunnel: w321 -> [w335 _]
          tunnel: [w334 w336] -> w320
          tunnel: w328 -> [w333 w337]
          tunnel: [w333 w337] -> _
          tunnel: w316 -> [_ w336]
          frame False {
            n301 = Decrement(x=w335) -> (x-1=w334:i32)
          }
          frame True {
          }
        }
        n302 = Path To String(path=w319) -> (string=w318:string)
        n303 = Index Array(array=w323, index=w320) -> (element=w327:string)
        n304 = Concatenate Strings(w318, "\\", w327) -> (w325:string)
        n305 = String To Path(string=w325) -> (path=w324:path)
        n306 = local write "Transfer File"(w324) -> ()
      }
      frame "Discard File" {
      }
      frame "Save" {
        n307 = stacked-sequence {
          seq-local: [w355 _] -> [_ w852]
          seq-local: [w354 _] -> [_ w850]
          tunnel: w346 -> [w356 w853]
          frame #0 {
            # "Saves each Re-calculated parameter in sequence"
            n308 = stacked-sequence {
              tunnel: [_ _ _ _ _ _ _ _ _ _ _ _ _ w820] -> w354
              tunnel: w356 -> [w376 _ _ _ _ _ _ _ _ _ _ _ _ _]
              frame #0 {
                n309 = call-poly <vilib>:"Read From Spreadsheet File.vi"("file path (dialog if empty)"=w376) -> ("all rows"=w375:string[][])  [unwired: 6 in, 4 out]
                n310 = Array Size(array=w375) -> (size(s)=w380:i32[])
                n311 = Array Subset(array=w375, index (row)=0, index (col)=0, length (col)=3) -> (w384:string[][])  [unwired: 1 in]
                n312 = Index Array(array=w380, index=0) -> (element=w378:i32)
                n313 = Reshape Array(w384, w378) -> (w377:string[])
                n314 = Search 1D Array(1D array=w377, element="Dielectric (nm):") -> (index of element=w387:i32)  [unwired: 1 in]
                n315 = Equal?(x=w387, y=-1) -> (x = y?=w386:bool)
                n316 = case shown="False" w386 {
                  tunnel: w375 -> [w395 w399]
                  tunnel: w387 -> [w391 _]
                  tunnel: [w390 w399] -> w385
                  frame False {
                    n317 = local read "Rec: Dielectric (d)"() -> (w397:dbl)
                    n318 = Number To Fractional String(number=w397) -> (F-format string=w392:string)  [unwired: 3 in]
                    n319 = Divide(x=w391, y=3) -> (x/y=w394:dbl)
                    n320 = To Word Integer(number=w394) -> (16bit integer=w393:i16)
                    n321 = Replace Array Subset(array=w395, new element=w392, index (row)=w393, index (col)=1) -> (w390:string[][])
                  }
                  frame True {
                  }
                }
                n322 = local write "Save Array"(w385) -> ()
              }
              frame #1 {
                n323 = local read "Save Array"() -> (w401:string[][])
                n324 = Array Size(array=w401) -> (size(s)=w404:i32[])
                n325 = Array Subset(array=w401, index (row)=0, index (col)=0, length (col)=3) -> (w408:string[][])  [unwired: 1 in]
                n326 = Index Array(array=w404, index=0) -> (element=w402:i32)
                n327 = Reshape Array(w408, w402) -> (w400:string[])
                n328 = Search 1D Array(1D array=w400, element="Comments:") -> (index of element=w411:i32)  [unwired: 1 in]
                n329 = Equal?(x=w411, y=-1) -> (x = y?=w410:bool)
                n330 = case shown="False" w410 {
                  tunnel: w401 -> [w419 w422]
                  tunnel: w411 -> [w416 _]
                  tunnel: [w415 w422] -> w409
                  frame False {
                    n331 = local read "New: Comments"() -> (w414:string)
                    n332 = Divide(x=w416, y=3) -> (x/y=w418:dbl)
                    n333 = To Word Integer(number=w418) -> (16bit integer=w417:i16)
                    n334 = Replace Array Subset(array=w419, new element=w414, index (row)=w417, index (col)=1) -> (w415:string[][])
                  }
                  frame True {
                  }
                }
                n335 = local write "Save Array"(w409) -> ()
              }
              frame #2 {
                n336 = local read "Save Array"() -> (w424:string[][])
                n337 = Array Size(array=w424) -> (size(s)=w427:i32[])
                n338 = Array Subset(array=w424, index (row)=0, index (col)=0, length (col)=3) -> (w431:string[][])  [unwired: 1 in]
                n339 = Index Array(array=w427, index=0) -> (element=w425:i32)
                n340 = Reshape Array(w431, w425) -> (w423:string[])
                n341 = Search 1D Array(1D array=w423, element="Length (um):") -> (index of element=w434:i32)  [unwired: 1 in]
                n342 = Equal?(x=w434, y=-1) -> (x = y?=w433:bool)
                n343 = case shown="False" w433 {
                  tunnel: w424 -> [w444 w447]
                  tunnel: w434 -> [w441 _]
                  tunnel: [w440 w447] -> w432
                  frame False {
                    n344 = local read "New: Length"() -> (w437:dbl)
                    n345 = Divide(x=w441, y=3) -> (x/y=w443:dbl)
                    n346 = Format Value(format string="%#g", value (0)=w437) -> (output string=w438:string)  [unwired: 1 in]
                    n347 = To Word Integer(number=w443) -> (16bit integer=w442:i16)
                    n348 = Replace Array Subset(array=w444, new element=w438, index (row)=w442, index (col)=1) -> (w440:string[][])
                  }
                  frame True {
                  }
                }
                n349 = local write "Save Array"(w432) -> ()
              }
              frame #3 {
                n350 = local read "Save Array"() -> (w449:string[][])
                n351 = Array Size(array=w449) -> (size(s)=w454:i32[])
                n352 = Array Subset(array=w449, index (row)=0, index (col)=0, length (col)=3) -> (w450:string[][])  [unwired: 1 in]
                n353 = Index Array(array=w454, index=0) -> (element=w456:i32)
                n354 = Reshape Array(w450, w456) -> (w448:string[])
                n355 = Search 1D Array(1D array=w448, element="Width (um):") -> (index of element=w459:i32)  [unwired: 1 in]
                n356 = Equal?(x=w459, y=-1) -> (x = y?=w458:bool)
                n357 = case shown="False" w458 {
                  tunnel: w459 -> [w467 _]
                  tunnel: w449 -> [w466 w472]
                  tunnel: [w465 w472] -> w457
                  frame False {
                    n358 = local read "New: Width"() -> (w462:dbl)
                    n359 = Divide(x=w467, y=3) -> (x/y=w469:dbl)
                    n360 = To Word Integer(number=w469) -> (16bit integer=w468:i16)
                    n361 = Format Value(format string="%#g", value (0)=w462) -> (output string=w463:string)  [unwired: 1 in]
                    n362 = Replace Array Subset(array=w466, new element=w463, index (row)=w468, index (col)=1) -> (w465:string[][])
                  }
                  frame True {
                  }
                }
                n363 = local write "Save Array"(w457) -> ()
              }
              frame #4 {
                w482 = "Sample Temp (K):"
                n364 = local read "Save Array"() -> (w474:string[][])
                n365 = Array Size(array=w474) -> (size(s)=w479:i32[])
                n366 = Array Subset(array=w474, index (row)=0, index (col)=0, length (col)=3) -> (w475:string[][])  [unwired: 1 in]
                n367 = Index Array(array=w479, index=0) -> (element=w481:i32)
                n368 = Reshape Array(w475, w481) -> (w473:string[])
                n369 = Search 1D Array(1D array=w473, element=w482) -> (index of element=w485:i32)  [unwired: 1 in]
                n370 = Equal?(x=w485, y=-1) -> (x = y?=w484:bool)
                n371 = case shown="False" w484 {
                  tunnel: w474 -> [w494 w508]
                  tunnel: w485 -> [w491 _]
                  tunnel: [w490 w507] -> w483
                  tunnel: w473 -> [_ w510]
                  tunnel: w482 -> [_ w497]
                  frame False {
                    n372 = local read "New: Temp"() -> (w488:dbl)
                    n373 = Divide(x=w491, y=3) -> (x/y=w493:dbl)
                    n374 = Format Value(format string="%#g", value (0)=w488) -> (output string=w487:string)  [unwired: 1 in]
                    n375 = To Word Integer(number=w493) -> (16bit integer=w492:i16)
                    n376 = Replace Array Subset(array=w494, new element=w487, index (row)=w492, index (col)=1) -> (w490:string[][])
                  }
                  frame True {
                    n377 = local read "New: Temp"() -> (w499:dbl)
                    n378 = Search 1D Array(1D array=w510, element="Width (um):") -> (index of element=w504:i32)  [unwired: 1 in]
                    n379 = Divide(x=w504, y=3) -> (x/y=w505:dbl)
                    n380 = To Word Integer(number=w505) -> (16bit integer=w503:i16)
                    n381 = Format Value(format string="%#g", value (0)=w499) -> (output string=w498:string)  [unwired: 1 in]
                    n382 = Build Array(w497, w498) -> (w501:string[])
                    n383 = Increment(x=w503) -> (x+1=w502:i16)
                    n384 = Insert Into Array(array=w508, index (row)=w502, new element=w501) -> (w507:string[][])  [unwired: 1 in]
                  }
                }
                n385 = local write "Save Array"(w483) -> ()
              }
              frame #5 {
                w520 = "Mobility-Sat (cm^2/Vs):"
                n386 = local read "Save Array"() -> (w512:string[][])
                n387 = Array Size(array=w512) -> (size(s)=w517:i32[])
                n388 = Array Subset(array=w512, index (row)=0, index (col)=0, length (col)=3) -> (w513:string[][])  [unwired: 1 in]
                n389 = Index Array(array=w517, index=0) -> (element=w519:i32)
                n390 = Reshape Array(w513, w519) -> (w511:string[])
                n391 = Search 1D Array(1D array=w511, element=w520) -> (index of element=w523:i32)  [unwired: 1 in]
                n392 = Equal?(x=w523, y=-1) -> (x = y?=w522:bool)
                n393 = case shown="False" w522 {
                  tunnel: w512 -> [w533 w543]
                  tunnel: w523 -> [w530 _]
                  tunnel: [w529 w542] -> w521
                  tunnel: w511 -> [_ w540]
                  tunnel: w520 -> [_ w538]
                  frame False {
                    n394 = local read "Re-Calculated Values Cluster"() -> (w526:T9)
                    n395 = Unbundle By Name(w526) -> ("Mobility-Sat"=w525:dbl)
                    n396 = Divide(x=w530, y=3) -> (x/y=w532:dbl)
                    n397 = To Word Integer(number=w532) -> (16bit integer=w531:i16)
                    n398 = Format Value(format string="%#g", value (0)=w525) -> (output string=w527:string)  [unwired: 1 in]
                    n399 = Replace Array Subset(array=w533, new element=w527, index (row)=w531, index (col)=1) -> (w529:string[][])
                  }
                  frame True {
                    n400 = local read "Re-Calculated Values Cluster"() -> (w537:T9)
                    n401 = Unbundle By Name(w537) -> ("Mobility-Sat"=w536:dbl)
                    n402 = Search 1D Array(1D array=w540, element="Mobility (cm^2/Vs):") -> (index of element=w546:i32)  [unwired: 1 in]
                    n403 = Divide(x=w546, y=3) -> (x/y=w547:dbl)
                    n404 = To Word Integer(number=w547) -> (16bit integer=w539:i16)
                    n405 = Format Value(format string="%#g", value (0)=w536) -> (output string=w541:string)  [unwired: 1 in]
                    n406 = Build Array(w538, w541) -> (w545:string[])
                    n407 = Replace Array Subset(array=w543, new element=w545, index (row)=w539) -> (w542:string[][])  [unwired: 1 in]
                  }
                }
                n408 = local write "Save Array"(w521) -> ()
              }
              frame #6 {
                w559 = "Mobility-Lin (cm^2/Vs):"
                n409 = local read "Save Array"() -> (w550:string[][])
                n410 = Array Size(array=w550) -> (size(s)=w556:i32[])
                n411 = Array Subset(array=w550, index (row)=0, index (col)=0, length (col)=3) -> (w552:string[][])  [unwired: 1 in]
                n412 = Index Array(array=w556, index=0) -> (element=w558:i32)
                n413 = Reshape Array(w552, w558) -> (w551:string[])
                n414 = Search 1D Array(1D array=w551, element=w559) -> (index of element=w562:i32)  [unwired: 1 in]
                n415 = Equal?(x=w562, y=-1) -> (x = y?=w561:bool)
                n416 = case shown="True" w561 {
                  tunnel: w550 -> [w572 w580]
                  tunnel: w562 -> [w569 _]
                  tunnel: [w568 w579] -> w560
                  tunnel: w551 -> [_ w578]
                  tunnel: w559 -> [_ w577]
                  frame False {
                    n417 = local read "Re-Calculated Values Cluster"() -> (w565:T9)
                    n418 = Unbundle By Name(w565) -> ("Moblitity-Lin"=w564:dbl)
                    n419 = Divide(x=w569, y=3) -> (x/y=w571:dbl)
                    n420 = To Word Integer(number=w571) -> (16bit integer=w570:i16)
                    n421 = Format Value(format string="%#g", value (0)=w564) -> (output string=w566:string)  [unwired: 1 in]
                    n422 = Replace Array Subset(array=w572, new element=w566, index (row)=w570, index (col)=1) -> (w568:string[][])
                  }
                  frame True {
                    n423 = local read "Re-Calculated Values Cluster"() -> (w576:T9)
                    n424 = Unbundle By Name(w576) -> ("Moblitity-Lin"=w575:dbl)
                    n425 = Search 1D Array(1D array=w578, element="Mobility-Sat (cm^2/Vs):") -> (index of element=w585:i32)  [unwired: 1 in]
                    n426 = Divide(x=w585, y=3) -> (x/y=w586:dbl)
                    n427 = To Word Integer(number=w586) -> (16bit integer=w584:i16)
                    n428 = Format Value(format string="%#g", value (0)=w575) -> (output string=w589:string)  [unwired: 1 in]
                    n429 = Build Array(w577, w589) -> (w582:string[])
                    n430 = Increment(x=w584) -> (x+1=w583:i16)
                    n431 = Insert Into Array(array=w580, index (row)=w583, new element=w582) -> (w579:string[][])  [unwired: 1 in]
                  }
                }
                n432 = local write "Save Array"(w560) -> ()
              }
              frame #7 {
                w599 = "On/Off I-Sat:"
                n433 = local read "Save Array"() -> (w590:string[][])
                n434 = Array Size(array=w590) -> (size(s)=w596:i32[])
                n435 = Array Subset(array=w590, index (row)=0, index (col)=0, length (col)=3) -> (w592:string[][])  [unwired: 1 in]
                n436 = Index Array(array=w596, index=0) -> (element=w598:i32)
                n437 = Reshape Array(w592, w598) -> (w591:string[])
                n438 = Search 1D Array(1D array=w591, element=w599) -> (index of element=w602:i32)  [unwired: 1 in]
                n439 = Equal?(x=w602, y=-1) -> (x = y?=w601:bool)
                n440 = case shown="True" w601 {
                  tunnel: w590 -> [w612 w621]
                  tunnel: w602 -> [w609 _]
                  tunnel: [w608 w622] -> w600
                  tunnel: w591 -> [_ w619]
                  tunnel: w599 -> [_ w617]
                  frame False {
                    n441 = local read "Re-Calculated Values Cluster"() -> (w605:T9)
                    n442 = Divide(x=w609, y=3) -> (x/y=w611:dbl)
                    n443 = Unbundle By Name(w605) -> ("On/Off"=w604:dbl)
                    n444 = To Word Integer(number=w611) -> (16bit integer=w610:i16)
                    n445 = Format Value(format string="%#g", value (0)=w604) -> (output string=w606:string)  [unwired: 1 in]
                    n446 = Replace Array Subset(array=w612, new element=w606, index (row)=w610, index (col)=1) -> (w608:string[][])
                  }
                  frame True {
                    n447 = local read "Re-Calculated Values Cluster"() -> (w616:T9)
                    n448 = Unbundle By Name(w616) -> ("On/Off"=w615:dbl)
                    n449 = Search 1D Array(1D array=w619, element="On/Off Current:") -> (index of element=w625:i32)  [unwired: 1 in]
                    n450 = Divide(x=w625, y=3) -> (x/y=w626:dbl)
                    n451 = To Word Integer(number=w626) -> (16bit integer=w618:i16)
                    n452 = Format Value(format string="%#g", value (0)=w615) -> (output string=w620:string)  [unwired: 1 in]
                    n453 = Build Array(w617, w620) -> (w624:string[])
                    n454 = Replace Array Subset(array=w621, new element=w624, index (row)=w618) -> (w622:string[][])  [unwired: 1 in]
                  }
                }
                n455 = local write "Save Array"(w600) -> ()
              }
              frame #8 {
                w638 = "Off I-Sat (A):"
                n456 = local read "Save Array"() -> (w629:string[][])
                n457 = Array Size(array=w629) -> (size(s)=w635:i32[])
                n458 = Array Subset(array=w629, index (row)=0, index (col)=0, length (col)=3) -> (w631:string[][])  [unwired: 1 in]
                n459 = Index Array(array=w635, index=0) -> (element=w637:i32)
                n460 = Reshape Array(w631, w637) -> (w630:string[])
                n461 = Search 1D Array(1D array=w630, element=w638) -> (index of element=w641:i32)  [unwired: 1 in]
                n462 = Equal?(x=w641, y=-1) -> (x = y?=w640:bool)
                n463 = case shown="True" w640 {
                  tunnel: w629 -> [w651 w659]
                  tunnel: w641 -> [w648 _]
                  tunnel: [w647 w658] -> w639
                  tunnel: w630 -> [_ w657]
                  tunnel: w638 -> [_ w656]
                  frame False {
                    n464 = local read "Re-Calculated Values Cluster"() -> (w644:T9)
                    n465 = Unbundle By Name(w644) -> ("Off Current"=w643:dbl)
                    n466 = Divide(x=w648, y=3) -> (x/y=w650:dbl)
                    n467 = Format Value(format string="%#g", value (0)=w643) -> (output string=w645:string)  [unwired: 1 in]
                    n468 = To Word Integer(number=w650) -> (16bit integer=w649:i16)
                    n469 = Replace Array Subset(array=w651, new element=w645, index (row)=w649, index (col)=1) -> (w647:string[][])
                  }
                  frame True {
                    n470 = local read "Re-Calculated Values Cluster"() -> (w655:T9)
                    n471 = Unbundle By Name(w655) -> ("Off Current"=w654:dbl)
                    n472 = Search 1D Array(1D array=w657, element="On/Off I-Sat:") -> (index of element=w664:i32)  [unwired: 1 in]
                    n473 = Divide(x=w664, y=3) -> (x/y=w665:dbl)
                    n474 = To Word Integer(number=w665) -> (16bit integer=w663:i16)
                    n475 = Format Value(format string="%#g", value (0)=w654) -> (output string=w668:string)  [unwired: 1 in]
                    n476 = Build Array(w656, w668) -> (w661:string[])
                    n477 = Increment(x=w663) -> (x+1=w662:i16)
                    n478 = Insert Into Array(array=w659, index (row)=w662, new element=w661) -> (w658:string[][])  [unwired: 1 in]
                  }
                }
                n479 = local write "Save Array"(w639) -> ()
              }
              frame #9 {
                w670 = "Vt-Sat (V):"
                n480 = local read "Save Array"() -> (w671:string[][])
                n481 = Array Size(array=w671) -> (size(s)=w676:i32[])
                n482 = Array Subset(array=w671, index (row)=0, index (col)=0, length (col)=3) -> (w672:string[][])  [unwired: 1 in]
                n483 = Index Array(array=w676, index=0) -> (element=w678:i32)
                n484 = Reshape Array(w672, w678) -> (w669:string[])
                n485 = Search 1D Array(1D array=w669, element=w670) -> (index of element=w681:i32)  [unwired: 1 in]
                n486 = Equal?(x=w681, y=-1) -> (x = y?=w680:bool)
                n487 = case shown="False" w680 {
                  tunnel: w671 -> [w690 w700]
                  tunnel: w681 -> [w686 _]
                  tunnel: [w685 w699] -> w679
                  tunnel: w670 -> [_ w698]
                  tunnel: w669 -> [_ w697]
                  frame False {
                    n488 = local read "Re-Calculated Values Cluster"() -> (w684:T9)
                    n489 = Unbundle By Name(w684) -> ("Vt-Sat"=w683:dbl)
                    n490 = Divide(x=w686, y=3) -> (x/y=w689:dbl)
                    n491 = To Word Integer(number=w689) -> (16bit integer=w688:i16)
                    n492 = Number To Fractional String(number=w683) -> (F-format string=w687:string)  [unwired: 3 in]
                    n493 = Replace Array Subset(array=w690, new element=w687, index (row)=w688, index (col)=1) -> (w685:string[][])
                  }
                  frame True {
                    n494 = local read "Re-Calculated Values Cluster"() -> (w694:T9)
                    n495 = Unbundle By Name(w694) -> ("Vt-Sat"=w693:dbl)
                    n496 = Search 1D Array(1D array=w697, element="Threshold V (V):") -> (index of element=w696:i32)  [unwired: 1 in]
                    n497 = Divide(x=w696, y=3) -> (x/y=w703:dbl)
                    n498 = To Word Integer(number=w703) -> (16bit integer=w695:i16)
                    n499 = Format Value(format string="%#g", value (0)=w693) -> (output string=w706:string)  [unwired: 1 in]
                    n500 = Build Array(w698, w706) -> (w702:string[])
                    n501 = Replace Array Subset(array=w700, new element=w702, index (row)=w695) -> (w699:string[][])  [unwired: 1 in]
                  }
                }
                n502 = local write "Save Array"(w679) -> ()
              }
              frame #10 {
                n503 = disable-structure shown="Disabled" {
                  frame Disabled {
                    n504 = local read "Save Array"() -> (w707:string[][])
                    n505 = Array Size(array=w707) -> (size(s)=w713:i32[])
                    n506 = Array Subset(array=w707, index (row)=0, index (col)=0, length (col)=3) -> (w709:string[][])  [unwired: 1 in]
                    n507 = Index Array(array=w713, index=0) -> (element=w715:i32)
                    n508 = Reshape Array(w709, w715) -> (w708:string[])
                    n509 = Search 1D Array(1D array=w708, element="VT-Lin (V):") -> (index of element=w718:i32)  [unwired: 1 in]
                    n510 = Equal?(x=w718, y=-1) -> (x = y?=w717:bool)
                    n511 = case shown="False" w717 {
                      tunnel: w707 -> [w727 w730]
                      tunnel: w718 -> [w724 _]
                      tunnel: [w723 w730] -> w716
                      frame False {
                        n512 = Divide(x=w724, y=3) -> (x/y=w726:dbl)
                        n513 = To Word Integer(number=w726) -> (16bit integer=w725:i16)
                        n514 = Format Value(format string="%#g") -> (output string=w721:string)  [unwired: 2 in]
                        n515 = Replace Array Subset(array=w727, new element=w721, index (row)=w725, index (col)=1) -> (w723:string[][])
                      }
                      frame True {
                      }
                    }
                    n516 = local write "Save Array"(w716) -> ()
                  }
                  frame Enabled {
                  }
                }
              }
              frame #11 {
                w731 = "STS-Sat (V/decade):"
                n517 = local read "Save Array"() -> (w733:string[][])
                n518 = Array Size(array=w733) -> (size(s)=w738:i32[])
                n519 = Array Subset(array=w733, index (row)=0, index (col)=0, length (col)=3) -> (w734:string[][])  [unwired: 1 in]
                n520 = Index Array(array=w738, index=0) -> (element=w740:i32)
                n521 = Reshape Array(w734, w740) -> (w732:string[])
                n522 = Search 1D Array(1D array=w732, element=w731) -> (index of element=w743:i32)  [unwired: 1 in]
                n523 = Equal?(x=w743, y=-1) -> (x = y?=w742:bool)
                n524 = case shown="True" w742 {
                  tunnel: w733 -> [w753 w761]
                  tunnel: w743 -> [w750 _]
                  tunnel: [w749 w762] -> w741
                  tunnel: w732 -> [_ w760]
                  tunnel: w731 -> [_ w759]
                  frame False {
                    n525 = local read "Re-Calculated Values Cluster"() -> (w745:T9)
                    n526 = Unbundle By Name(w745) -> ("STS"=w746:dbl)
                    n527 = Divide(x=w750, y=3) -> (x/y=w752:dbl)
                    n528 = To Word Integer(number=w752) -> (16bit integer=w751:i16)
                    n529 = Format Value(format string="%#g", value (0)=w746) -> (output string=w747:string)  [unwired: 1 in]
                    n530 = Replace Array Subset(array=w753, new element=w747, index (row)=w751, index (col)=1) -> (w749:string[][])
                  }
                  frame True {
                    n531 = local read "Re-Calculated Values Cluster"() -> (w756:T9)
                    n532 = Unbundle By Name(w756) -> ("STS"=w757:dbl)
                    n533 = Search 1D Array(1D array=w760, element="S.T.S. (V/decade):") -> (index of element=w765:i32)  [unwired: 1 in]
                    n534 = Divide(x=w765, y=3) -> (x/y=w766:dbl)
                    n535 = To Word Integer(number=w766) -> (16bit integer=w758:i16)
                    n536 = Format Value(format string="%#g", value (0)=w757) -> (output string=w769:string)  [unwired: 1 in]
                    n537 = Build Array(w759, w769) -> (w764:string[])
                    n538 = Replace Array Subset(array=w761, new element=w764, index (row)=w758) -> (w762:string[][])  [unwired: 1 in]
                  }
                }
                n539 = local write "Save Array"(w741) -> ()
              }
              frame #12 {
                w770 = "Trap Density-VT (Traps/Vcm^2):"
                n540 = local read "Save Array"() -> (w772:string[][])
                n541 = Array Size(array=w772) -> (size(s)=w777:i32[])
                n542 = Array Subset(array=w772, index (row)=0, index (col)=0, length (col)=3) -> (w773:string[][])  [unwired: 1 in]
                n543 = Index Array(array=w777, index=0) -> (element=w779:i32)
                n544 = Reshape Array(w773, w779) -> (w771:string[])
                n545 = Search 1D Array(1D array=w771, element=w770) -> (index of element=w782:i32)  [unwired: 1 in]
                n546 = Equal?(x=w782, y=-1) -> (x = y?=w781:bool)
                n547 = case shown="True" w781 {
                  tunnel: w772 -> [w792 w799]
                  tunnel: w782 -> [w788 _]
                  tunnel: [w787 w800] -> w780
                  tunnel: w771 -> [_ w798]
                  tunnel: w770 -> [_ w797]
                  frame False {
                    n548 = local read "Re-Calculated Values Cluster"() -> (w785:T9)
                    n549 = Unbundle By Name(w785) -> ("Trap Density-VT"=w784:dbl)
                    n550 = Divide(x=w788, y=3) -> (x/y=w791:dbl)
                    n551 = To Word Integer(number=w791) -> (16bit integer=w790:i16)
                    n552 = Format Value(format string="%#g", value (0)=w784) -> (output string=w789:string)  [unwired: 1 in]
                    n553 = Replace Array Subset(array=w792, new element=w789, index (row)=w790, index (col)=1) -> (w787:string[][])
                  }
                  frame True {
                    n554 = local read "Re-Calculated Values Cluster"() -> (w796:T9)
                    n555 = Unbundle By Name(w796) -> ("Trap Density-VT"=w795:dbl)
                    n556 = Search 1D Array(1D array=w798, element="STS-Sat (V/decade):") -> (index of element=w805:i32)  [unwired: 1 in]
                    n557 = Divide(x=w805, y=3) -> (x/y=w804:dbl)
                    n558 = To Word Integer(number=w804) -> (16bit integer=w806:i16)
                    n559 = Format Value(format string="%#g", value (0)=w795) -> (output string=w801:string)  [unwired: 1 in]
                    n560 = Build Array(w797, w801) -> (w808:string[])
                    n561 = Increment(x=w806) -> (x+1=w807:i16)
                    n562 = Insert Into Array(array=w799, index (row)=w807, new element=w808) -> (w800:string[][])  [unwired: 1 in]
                  }
                }
                n563 = local write "Save Array"(w780) -> ()
              }
              frame #13 {
                w810 = "Trap Density-STS (Traps/Vcm^2):"
                n564 = local read "Save Array"() -> (w812:string[][])
                n565 = Array Size(array=w812) -> (size(s)=w817:i32[])
                n566 = Array Subset(array=w812, index (row)=0, index (col)=0, length (col)=3) -> (w813:string[][])  [unwired: 1 in]
                n567 = Index Array(array=w817, index=0) -> (element=w819:i32)
                n568 = Reshape Array(w813, w819) -> (w811:string[])
                n569 = Search 1D Array(1D array=w811, element=w810) -> (index of element=w822:i32)  [unwired: 1 in]
                n570 = Equal?(x=w822, y=-1) -> (x = y?=w821:bool)
                n571 = case shown="True" w821 {
                  tunnel: w812 -> [w832 w839]
                  tunnel: w822 -> [w829 _]
                  tunnel: [w828 w840] -> w820
                  tunnel: w811 -> [_ w838]
                  tunnel: w810 -> [_ w837]
                  frame False {
                    n572 = local read "Re-Calculated Values Cluster"() -> (w825:T9)
                    n573 = Unbundle By Name(w825) -> ("Trap Density-STS"=w824:dbl)
                    n574 = Divide(x=w829, y=3) -> (x/y=w831:dbl)
                    n575 = To Word Integer(number=w831) -> (16bit integer=w830:i16)
                    n576 = Format Value(format string="%#g", value (0)=w824) -> (output string=w826:string)  [unwired: 1 in]
                    n577 = Replace Array Subset(array=w832, new element=w826, index (row)=w830, index (col)=1) -> (w828:string[][])
                  }
                  frame True {
                    n578 = local read "Re-Calculated Values Cluster"() -> (w836:T9)
                    n579 = Unbundle By Name(w836) -> ("Trap Density-STS"=w835:dbl)
                    n580 = Search 1D Array(1D array=w838, element="Trap Density-VT (Traps/Vcm^2):") -> (index of element=w845:i32)  [unwired: 1 in]
                    n581 = Divide(x=w845, y=3) -> (x/y=w846:dbl)
                    n582 = To Word Integer(number=w846) -> (16bit integer=w844:i16)
                    n583 = Format Value(format string="%#g", value (0)=w835) -> (output string=w849:string)  [unwired: 1 in]
                    n584 = Build Array(w837, w849) -> (w842:string[])
                    n585 = Increment(x=w844) -> (x+1=w843:i16)
                    n586 = Insert Into Array(array=w839, index (row)=w843, new element=w842) -> (w840:string[][])  [unwired: 1 in]
                  }
                }
                n587 = local write "Save Array"(w820) -> ()
              }
            }
            n588 = local read "New: Temp"() -> (w357:dbl)
            n589 = local read "New: Width"() -> (w358:dbl)
            n590 = local read "New: Length"() -> (w360:dbl)
            n591 = local read "Index"() -> (w359:string)
            n592 = To Single Precision Float(number=w357) -> (single precision float=w374:sgl)
            n593 = Number To Decimal String(number=w374) -> (decimal integer string=w369:string)  [unwired: 1 in]
            n594 = To Single Precision Float(number=w358) -> (single precision float=w373:sgl)
            n595 = To Single Precision Float(number=w360) -> (single precision float=w372:sgl)
            n596 = Strip Path(path=w356) -> (stripped path=w361:path)  [unwired: 1 out]
            n597 = Number To Decimal String(number=w372) -> (decimal integer string=w367:string)  [unwired: 1 in]
            n598 = Number To Decimal String(number=w373) -> (decimal integer string=w366:string)  [unwired: 1 in]
            n599 = Concatenate Strings("_", w369, "K") -> (w371:string)
            n600 = call "Build Text"("Temp"=w371, "Index"=w359, "Length"=w367, "Width"=w366) -> ("Result"=w365:string)  [unwired: 10 in, 1 out]
            n601 = Path To String(path=w361) -> (string=w363:string)
            n602 = Concatenate Strings(w363, "\\", w365) -> (w364:string)
            n603 = String To Path(string=w364) -> (path=w355:path)
          }
          frame #1 {
            n604 = flat-sequence {
              tunnel: w853 -> [w855]
              tunnel: w852 -> [w854]
              tunnel: [w854] -> w851
              tunnel: w851 -> [w861]
              tunnel: w850 -> [w860]
              frame #0 {
                n605 = Equal?(x=w855, y=w854) -> (x = y?=w856:bool)
                n606 = case shown="False" w856 {
                  tunnel: w855 -> [w859 _]
                  tunnel: w854 -> [w858 _]
                  frame False {
                    n607 = Move(source path=w859, 9:TRUE, 10:w858) -> ()  [unwired: 2 in, 3 out]
                  }
                  frame True {
                  }
                }
              }
              frame #1 {
                n608 = local write "Transfer File"(w861) -> ()
                n609 = call-poly <vilib>:"Write To Spreadsheet File.vi"("2D data"=w860, "file path (dialog if empty)"=w861) -> ()  [unwired: 6 in, 1 out]
              }
            }
          }
        }
        n610 = Cluster To Array(cluster=w345) -> (array=w344:bool[])
        n611 = Boolean Array To Number(Boolean array=w344) -> (number=w343:u32)
        n612 = Equal To 0?(x=w343) -> (x = 0?=w342:bool)
        n613 = case shown="True" w342 {
          tunnel: [MegaAwesome_States."Read Data" w349] -> w341
          tunnel: w340 -> [_ w353]
          frame False {
          }
          frame True {
            n614 = Unbundle By Name(w353) -> ("Save Next"=w352:bool)
            n615 = Select(t=MegaAwesome_States."No Event", s=w352, f=MegaAwesome_States."Next File") -> (s? t:f=w349:T2)
          }
        }
      }
      frame "Exit" {
      }
      frame "Save Lines" {
      }
      frame "Export" {
        n616 = flat-sequence {
          frame #0 {
            n617 = stacked-sequence {
              frame #0 {
                n618 = local read "Independant Variable:"() -> (w868:string)
                n619 = Equal?(x=w868, y="Length (um):") -> (x = y?=w869:bool)
                n620 = case shown="True" w869 {
                  frame False {
                  }
                  frame True {
                    n621 = local write "X Axis Display Type"("1") -> ()
                    n622 = local write "Opj X Axis"("2") -> ()
                  }
                }
              }
              frame #1 {
                n623 = local read "Independant Variable:"() -> (w873:string)
                n624 = Equal?(x=w873, y="Sample Temp (K):") -> (x = y?=w874:bool)
                n625 = case shown="True" w874 {
                  frame False {
                  }
                  frame True {
                    n626 = local write "X Axis Display Type"("1") -> ()
                    n627 = local write "Opj X Axis"("1") -> ()
                  }
                }
              }
              frame #2 {
                n628 = local read "Independant Variable:"() -> (w878:string)
                n629 = Equal?(x=w878, y="Mobility-Sat (cm^2/Vs):") -> (x = y?=w879:bool)
                n630 = case shown="True" w879 {
                  frame False {
                  }
                  frame True {
                    n631 = local write "X Axis Display Type"("2") -> ()
                    n632 = local write "Opj X Axis"("2") -> ()
                  }
                }
              }
              frame #3 {
                n633 = local read "Independant Variable:"() -> (w883:string)
                n634 = Equal?(x=w883, y="Mobility-Lin (cm^2/Vs):") -> (x = y?=w884:bool)
                n635 = case shown="True" w884 {
                  frame False {
                  }
                  frame True {
                    n636 = local write "X Axis Display Type"("2") -> ()
                    n637 = local write "Opj X Axis"("2") -> ()
                  }
                }
              }
              frame #4 {
                n638 = local read "Independant Variable:"() -> (w888:string)
                n639 = Equal?(x=w888, y="On/Off I-Sat:") -> (x = y?=w889:bool)
                n640 = case shown="True" w889 {
                  frame False {
                  }
                  frame True {
                    n641 = local write "X Axis Display Type"("2") -> ()
                    n642 = local write "Opj X Axis"("2") -> ()
                  }
                }
              }
              frame #5 {
                n643 = local read "Independant Variable:"() -> (w893:string)
                n644 = Equal?(x=w893, y="Off I-Sat (A):") -> (x = y?=w894:bool)
                n645 = case shown="True" w894 {
                  frame False {
                  }
                  frame True {
                    n646 = local write "X Axis Display Type"("2") -> ()
                    n647 = local write "Opj X Axis"("2") -> ()
                  }
                }
              }
              frame #6 {
                n648 = local read "Independant Variable:"() -> (w898:string)
                n649 = Equal?(x=w898, y="Vt-Sat (V):") -> (x = y?=w899:bool)
                n650 = case shown="True" w899 {
                  frame False {
                  }
                  frame True {
                    n651 = local write "X Axis Display Type"("1") -> ()
                    n652 = local write "Opj X Axis"("1") -> ()
                  }
                }
              }
              frame #7 {
                n653 = local read "Independant Variable:"() -> (w903:string)
                n654 = Equal?(x=w903, y="STS-Sat (V/decade):") -> (x = y?=w904:bool)
                n655 = case shown="True" w904 {
                  frame False {
                  }
                  frame True {
                    n656 = local write "X Axis Display Type"("1") -> ()
                    n657 = local write "Opj X Axis"("1") -> ()
                  }
                }
              }
              frame #8 {
                n658 = local read "Independant Variable:"() -> (w908:string)
                n659 = Equal?(x=w908, y="Trap Density-VT (Traps/Vcm^2):") -> (x = y?=w909:bool)
                n660 = case shown="True" w909 {
                  frame False {
                  }
                  frame True {
                    n661 = local write "X Axis Display Type"("2") -> ()
                    n662 = local write "Opj X Axis"("2") -> ()
                  }
                }
              }
              frame #9 {
                n663 = local read "Independant Variable:"() -> (w913:string)
                n664 = Equal?(x=w913, y="Trap Density-STS (Traps/Vcm^2):") -> (x = y?=w914:bool)
                n665 = case shown="True" w914 {
                  frame False {
                  }
                  frame True {
                    n666 = local write "X Axis Display Type"("2") -> ()
                    n667 = local write "Opj X Axis"("2") -> ()
                  }
                }
              }
            }
          }
          frame #1 {
            n668 = local read "Transfer Folder"() -> (w922:path)
            n669 = Build Path(base path=w922, name or relative path="Stats") -> (appended path=w923:path)
            n670 = local read "Origin Project File"() -> (w934:path)
            n671 = call <vilib>:"Check if File or Folder Exists.vi"("path"=w923) -> ("file or folder exists?"=w938:bool, "dup path"=w937:path)  [unwired: 8 in, 1 out]
            n672 = call <userlib>:"OA_ConnectToOrigin.vi"() -> ("error out"=w935:errorcluster, "Origin.IOApplication"=w936:refnum<k7>)  [unwired: 8 in]
            n673 = case shown="False" w938 {
              tunnel: w937 -> [w1111 w1112]
              tunnel: [w1110 w1112] -> w921
              frame False {
                n674 = Create Folder(path (use dialog)=w1111) -> (created path=w1110:path)  [unwired: 2 in, 2 out]
              }
              frame True {
              }
            }
            n675 = call "File Dialog"("start path"=w923) -> ("selected path"=w925:path)  [unwired: 11 in, 3 out]
            n676 = call <userlib>:"OA_Load.vi"("error in (no error)"=w935, "Path"=w934, "Origin.IOApplication"=w936) -> ("error out"=w932:errorcluster, "Origin.IOApplication"=w933:refnum<k7>)  [unwired: 1 out]
            n677 = call "OAExecute.vi"("script"="document -m 3;", "Error IO"=w932, "Origin.IOApplication"=w933) -> ("Error IO Out"=w930:errorcluster, "Origin.IOApplication"=w931:refnum<k7>)  [unwired: 1 in, 1 out]
            n678 = local read "Independant Variable:"() -> (w918:string)
            n679 = stacked-sequence {
              tunnel: w922 -> [w949 w979 w991 w1013 w1033 w1054 w1075 w1098]
              tunnel: w921 -> [w950 w978 w992 w1012 w1034 w1055 w1076 w1099]
              tunnel: w931 -> [w952 w976 w994 w1015 w1036 w1057 w1078 w1101]
              tunnel: w930 -> [w951 w977 w993 w1014 w1035 w1056 w1077 w1100]
              tunnel: [_ _ _ _ _ _ _ w1096] -> w920
              tunnel: [_ _ _ _ _ _ _ w1097] -> w919
              tunnel: w918 -> [w948 w969 w990 w1011 w1032 w1053 w1074 w1095]
              frame #0 {
                n680 = local read "X Axis Display Type"() -> (w940:string)
                n681 = local read "Opj X Axis"() -> (w945:string)
                n682 = Concatenate Strings("window -a MOBLGraph;\nlayer.x.type=", w945, "; layer.x.label.numFormat = ", w940, "; Y3 = 1; X3 = 1;", "window -a MOBLTable;\nwindow -s TV;") -> (w943:string)
                n683 = call "Param_Analysis_7_24b_JW.vi"("Independant Variable"=w948, "error in (no error)"=w951, "Data Folder"=w949, "Parameter String"="Mobility-Lin (cm^2/Vs):", "Parameter Name"="Mobility-Lin", "Stats Folder"=w950) -> ("error out"=w954:errorcluster, "Output Array"=w956:string[][], "Variables"=w947:T16)  [unwired: 2 in, 1 out]
                n684 = call "Origin_Export_7_27a_JW.vi"("Input Conditions"=w947, "Analysis Array"=w956, "error in (no error)"=w954, "Parameter Worksheet Name"="[MOBLTable]Mobilities", "Parameter Folder Script"="pe_cd \"Mobility-Lin\";", "Origin.IOApplication"=w952) -> ("error out"=w953:errorcluster, "reference out"=w955:refnum<k7>)  [unwired: 3 in, 1 out]
                n685 = call "OAExecute.vi"("script"=w943, "Error IO"=w953, "Origin.IOApplication"=w955) -> ()  [unwired: 1 in, 3 out]
              }
              frame #1 {
                n686 = local read "X Axis Display Type"() -> (w961:string)
                n687 = local read "Opj X Axis"() -> (w966:string)
                n688 = Concatenate Strings("window -a MOBSGraph;\nlayer.x.type=", w966, "; layer.x.label.numFormat = ", w961, "; Y3 = 1; X3 = 1;", "window -a MOBSTable;\nwindow -s TV;") -> (w964:string)
                n689 = call "Param_Analysis_7_24b_JW.vi"("Independant Variable"=w969, "error in (no error)"=w977, "Data Folder"=w979, "Parameter String"="Mobility-Sat (cm^2/Vs):", "Parameter Name"="Mobility-Sat", "Stats Folder"=w978) -> ("error out"=w972:errorcluster, "Output Array"=w970:string[][], "Variables"=w968:T16)  [unwired: 2 in, 1 out]
                n690 = call "Origin_Export_7_27a_JW.vi"("Input Conditions"=w968, "Analysis Array"=w970, "error in (no error)"=w972, "Parameter Worksheet Name"="[MOBSTable]Mobilities", "Parameter Folder Script"="pe_cd \"Mobility-Sat\";", "Origin.IOApplication"=w976) -> ("error out"=w971:errorcluster, "reference out"=w973:refnum<k7>)  [unwired: 3 in, 1 out]
                n691 = call "OAExecute.vi"("script"=w964, "Error IO"=w971, "Origin.IOApplication"=w973) -> ()  [unwired: 1 in, 3 out]
              }
              frame #2 {
                n692 = local read "X Axis Display Type"() -> (w982:string)
                n693 = local read "Opj X Axis"() -> (w987:string)
                n694 = Concatenate Strings("window -a NSTSGraph;\nlayer.x.type=", w987, "; layer.x.label.numFormat = ", w982, "; Y3 = 1; X3 = 1;", "window -a NSTSTable;\nwindow -s TV;") -> (w985:string)
                n695 = call "Param_Analysis_7_24b_JW.vi"("Independant Variable"=w990, "error in (no error)"=w993, "Data Folder"=w991, "Parameter String"="Trap Density-STS (Traps/Vcm^2):", "Parameter Name"="Trap Density-STS", "Stats Folder"=w992) -> ("error out"=w997:errorcluster, "Output Array"=w995:string[][], "Variables"=w989:T16)  [unwired: 2 in, 1 out]
                n696 = call "Origin_Export_7_27a_JW.vi"("Input Conditions"=w989, "Analysis Array"=w995, "error in (no error)"=w997, "Parameter Worksheet Name"="[NSTSTable]Trap Densities", "Parameter Folder Script"="pe_cd \"N-STS\";", "Origin.IOApplication"=w994) -> ("error out"=w996:errorcluster, "reference out"=w998:refnum<k7>)  [unwired: 3 in, 1 out]
                n697 = call "OAExecute.vi"("script"=w985, "Error IO"=w996, "Origin.IOApplication"=w998) -> ()  [unwired: 1 in, 3 out]
              }
              frame #3 {
                n698 = local read "X Axis Display Type"() -> (w1003:string)
                n699 = local read "Opj X Axis"() -> (w1008:string)
                n700 = call "Param_Analysis_7_24b_JW.vi"("Independant Variable"=w1011, "error in (no error)"=w1014, "Data Folder"=w1013, "Parameter String"="Trap Density-VT (Traps/Vcm^2):", "Parameter Name"="Trap Density-Vt", "Stats Folder"=w1012) -> ("error out"=w1018:errorcluster, "Output Array"=w1016:string[][], "Variables"=w1010:T16)  [unwired: 2 in, 1 out]
                n701 = Concatenate Strings("window -a NVtGraph;\nlayer.x.type=", w1008, "; layer.x.label.numFormat = ", w1003, "; Y3 = 1; X3 = 1;", "window -a NVtTable;\nwindow -s TV;") -> (w1006:string)
                n702 = call "Origin_Export_7_27a_JW.vi"("Input Conditions"=w1010, "Analysis Array"=w1016, "error in (no error)"=w1018, "Parameter Worksheet Name"="[NVTTable]Trap Densities", "Parameter Folder Script"="pe_cd \"N-Vt\";", "Origin.IOApplication"=w1015) -> ("error out"=w1017:errorcluster, "reference out"=w1019:refnum<k7>)  [unwired: 3 in, 1 out]
                n703 = call "OAExecute.vi"("script"=w1006, "Error IO"=w1017, "Origin.IOApplication"=w1019) -> ()  [unwired: 1 in, 3 out]
              }
              frame #4 {
                n704 = local read "X Axis Display Type"() -> (w1024:string)
                n705 = local read "Opj X Axis"() -> (w1029:string)
                n706 = Concatenate Strings("window -a OffIGraph;\nlayer.x.type=", w1029, "; layer.x.label.numFormat = ", w1024, "; Y3 = 1; X3 = 1;", "window -a OffITable;\nwindow -s TV;") -> (w1027:string)
                n707 = call "Param_Analysis_7_24b_JW.vi"("Independant Variable"=w1032, "error in (no error)"=w1035, "Data Folder"=w1033, "Parameter String"="Off I-Sat (A):", "Parameter Name"="Off I-Sat", "Stats Folder"=w1034) -> ("error out"=w1039:errorcluster, "Output Array"=w1037:string[][], "Variables"=w1031:T16)  [unwired: 2 in, 1 out]
                n708 = call "Origin_Export_7_27a_JW.vi"("Input Conditions"=w1031, "Analysis Array"=w1037, "error in (no error)"=w1039, "Parameter Worksheet Name"="[OffItable]OffCurrents", "Parameter Folder Script"="pe_cd \"OffI-Sat\";", "Origin.IOApplication"=w1036) -> ("error out"=w1038:errorcluster, "reference out"=w1040:refnum<k7>)  [unwired: 3 in, 1 out]
                n709 = call "OAExecute.vi"("script"=w1027, "Error IO"=w1038, "Origin.IOApplication"=w1040) -> ()  [unwired: 1 in, 3 out]
              }
              frame #5 {
                n710 = local read "X Axis Display Type"() -> (w1045:string)
                n711 = local read "Opj X Axis"() -> (w1050:string)
                n712 = Concatenate Strings("window -a OnOffGraph;\nlayer.x.type=", w1050, "; layer.x.label.numFormat = ", w1045, "; Y3 = 1; X3 = 1;", "window -a OnOffTable;\nwindow -s TV;") -> (w1048:string)
                n713 = call "Param_Analysis_7_24b_JW.vi"("Independant Variable"=w1053, "error in (no error)"=w1056, "Data Folder"=w1054, "Parameter String"="On/Off I-Sat:", "Parameter Name"="OnOff Ratio", "Stats Folder"=w1055) -> ("error out"=w1060:errorcluster, "Output Array"=w1058:string[][], "Variables"=w1052:T16)  [unwired: 2 in, 1 out]
                n714 = call "Origin_Export_7_27a_JW.vi"("Input Conditions"=w1052, "Analysis Array"=w1058, "error in (no error)"=w1060, "Parameter Worksheet Name"="[OnOffTable]On/Off Ratios", "Parameter Folder Script"="pe_cd \"OnOff-Ratio\";", "Origin.IOApplication"=w1057) -> ("error out"=w1059:errorcluster, "reference out"=w1061:refnum<k7>)  [unwired: 3 in, 1 out]
                n715 = call "OAExecute.vi"("script"=w1048, "Error IO"=w1059, "Origin.IOApplication"=w1061) -> ()  [unwired: 1 in, 3 out]
              }
              frame #6 {
                n716 = local read "X Axis Display Type"() -> (w1066:string)
                n717 = local read "Opj X Axis"() -> (w1071:string)
                n718 = call "Param_Analysis_7_24b_JW.vi"("Independant Variable"=w1074, "error in (no error)"=w1077, "Data Folder"=w1075, "Parameter String"="STS-Sat (V/decade):", "Parameter Name"="STS-Sat", "Stats Folder"=w1076) -> ("error out"=w1081:errorcluster, "Output Array"=w1079:string[][], "Variables"=w1073:T16)  [unwired: 2 in, 1 out]
                n719 = Concatenate Strings("window -a SGraph;\nlayer.x.type=", w1071, "; layer.x.label.numFormat = ", w1066, "; Y3 = 1; X3 = 1;", "window -a STable;\nwindow -s TV;") -> (w1069:string)
                n720 = call "Origin_Export_7_27a_JW.vi"("Input Conditions"=w1073, "Analysis Array"=w1079, "error in (no error)"=w1081, "Parameter Worksheet Name"="[STable]Threshold Swing", "Parameter Folder Script"="pe_cd \"STS-Sat\";", "Origin.IOApplication"=w1078) -> ("error out"=w1080:errorcluster, "reference out"=w1082:refnum<k7>)  [unwired: 3 in, 1 out]
                n721 = call "OAExecute.vi"("script"=w1069, "Error IO"=w1080, "Origin.IOApplication"=w1082) -> ()  [unwired: 1 in, 3 out]
              }
              frame #7 {
                n722 = local read "X Axis Display Type"() -> (w1087:string)
                n723 = local read "Opj X Axis"() -> (w1092:string)
                n724 = Concatenate Strings("window -a VtGraph;\nlayer.x.type=", w1092, "; layer.x.label.numFormat = ", w1087, "; Y3 = 1; X3 = 1;", "window -a VtTable;\nwindow -s TV;") -> (w1090:string)
                n725 = call "Param_Analysis_7_24b_JW.vi"("Independant Variable"=w1095, "error in (no error)"=w1100, "Data Folder"=w1098, "Parameter String"="Vt-Sat (V):", "Parameter Name"="Vt-Sat", "Stats Folder"=w1099) -> ("error out"=w1104:errorcluster, "Output Array"=w1102:string[][], "Variables"=w1094:T16)  [unwired: 2 in, 1 out]
                n726 = call "Origin_Export_7_27a_JW.vi"("Input Conditions"=w1094, "Analysis Array"=w1102, "error in (no error)"=w1104, "Parameter Worksheet Name"="[VtTable]Threshold Voltages", "Parameter Folder Script"="pe_cd \"Vt-Sat\";", "Origin.IOApplication"=w1101) -> ("error out"=w1103:errorcluster, "reference out"=w1105:refnum<k7>)  [unwired: 3 in, 1 out]
                n727 = call "OAExecute.vi"("script"=w1090, "Error IO"=w1103, "Origin.IOApplication"=w1105) -> ("Error IO Out"=w1096:errorcluster, "Origin.IOApplication"=w1097:refnum<k7>)  [unwired: 1 in, 1 out]
              }
            }
            n728 = Path To String(path=w925) -> (string=w924:string)
            n729 = call "OAExecute.vi"("script"="pe_cd /; ", "Error IO"=w920, "Origin.IOApplication"=w919) -> ("Error IO Out"=w926:errorcluster, "Origin.IOApplication"=w927:refnum<k7>)  [unwired: 1 in, 1 out]
            n730 = call <userlib>:"OASaveProject.vi"("path"=w924, "Error IO"=w926, "Origin.IOApplication"=w927) -> ()  [unwired: 3 out]
          }
        }
      }
    }
    "Current State" <- w13
    "Folder Index" <- w6
    n731 = Equal?(x=w15, y=MegaAwesome_States."Exit") -> (x = y?=w16:bool)
    n732 = Wait (ms)(milliseconds to wait=10) -> ()  [unwired: 1 out]
  }
